vi "1_VisualAD_Train_Eval_Investigate.vi"(0 "NNFE_Paths":T1={"CFG"=path "D:/Ngene/GitHub/deepltk_examples/3_Image_Processing/36_Anomaly_Detection/NNFE/WRN_50_2_2_L3/WRN_50_2_2_BBoneL3.cfg", "BIN"=path "D:/Ngene/GitHub/deepltk_examples/3_Image_Processing/36_Anomaly_Detection/NNFE/WRN_50_2_2_L3/WRN_50_2_2_BBoneL3.bin"}, 1 "Dest. Path":path=path "D:/Ngene/GitHub/deepltk_examples/3_Image_Processing/36_Anomaly_Detection/Models", 2 "Dataset_Path(Train)":path=path "D:/Ngene/GitHub/deepltk_examples/3_Image_Processing/36_Anomaly_Detection/Dataset/Playing_Cards_3ofHearts/train", 3 "Dataset_Path(Validation)":path=path "D:/Ngene/GitHub/deepltk_examples/3_Image_Processing/36_Anomaly_Detection/Dataset/Playing_Cards_3ofHearts/test", 4 "Ground_Truth_Folder_Path":path, 5 "error in":errorcluster, 6 "NNFE CFG":T7={"Name"="Cards_3ofHearts", "Layer_Selection_By"=enum."Stride", "Feature_Layers"={"[LayerID, PatchSize]"=[{"Layer_ID"=8, "Patch_Size"=3}]}, "Interpolation_Type"=enum."Bi-Linear"}, 7 "Dim_Reduction":T11={"Method"=enum."None", "Target_Dim"=-1, "Seed"=42}, 8 "NNPC_Setup":T2={"Input_Dims"={"C"=3, "H"=320, "W"=320}, "mBatch"=1, "Device"=enum."GPU", "GPU Id"=0}, 9 "CoreSet_Params":T5={"Distance_Metric"=enum."Euclidean", "CoreSet_Size"=2000.0, "Start_idx"=3}) -> (11 "MemBank Size":i32=2000, 13 "dT_Total":dbl=4.467676200001733 format="%.2f", 14 "Model Paths":T1={"CFG"=path "D:/Ngene/GitHub/deepltk_examples/3_Image_Processing/36_Anomaly_Detection/Models/NNPC_Cards_3ofHearts__25_10_21__19_21_13/NNPC_Cards_3ofHearts_25_10_21__19_21_13.cfg", "BIN"=path "D:/Ngene/GitHub/deepltk_examples/3_Image_Processing/36_Anomaly_Detection/Models/NNPC_Cards_3ofHearts__25_10_21__19_21_13/NNPC_Cards_3ofHearts_25_10_21__19_21_13.bin"}, 15 "Evaluation Metrics":T13={"Evaluation_Metrics(Pixel)"={"Scores(Good)"={"X Values"=[4.812818005084992, 5.126218183040619, 5.4396183609962465, 5.753018538951874, 6.066418716907501, 6.379818894863129, 6.693219072818756, 7.006619250774383, 7.320019428730012, 7.633419606685639, 7.946819784641266, 8.260219962596892, 8.57362014055252, 8.88702031850815, 9.200420496463774, 9.513820674419403, 9.827220852375032, 10.14062103033066, 10.454021208286285, 10.767421386241914, 11.080821564197542, 11.394221742153167, 11.707621920108796, 12.021022098064424, 12.33442227602005, 12.647822453975678, 12.961222631931307, 13.274622809886932, 13.58802298784256, 13.901423165798189, 14.214823343753816, 14.528223521709442, 14.841623699665071, 15.155023877620698, 15.468424055576325, 15.781824233531953, 16.095224411487578, 16.408624589443207, 16.722024767398835, 17.035424945354464, 17.348825123310093, 17.662225301265718, 17.975625479221343, 18.28902565717697, 18.6024258351326, 18.91582601308823, 19.229226191043857, 19.542626368999485, 19.856026546955107, 20.169426724910736, 20.482826902866364, 20.796227080821993, 21.10962725877762, 21.423027436733246, 21.736427614688875, 22.0498277926445, 22.36322797060013, 22.676628148555757, 22.990028326511386, 23.303428504467014, 23.61682868242264, 23.930228860378268, 24.243629038333893, 24.55702921628952, 24.87042939424515, 25.18382957220078, 25.497229750156404, 25.810629928112032, 26.124030106067657, 26.437430284023286, 26.750830461978914, 27.064230639934543, 27.37763081789017, 27.691030995845797, 28.004431173801425, 28.31783135175705, 28.63123152971268, 28.944631707668307, 29.258031885623936, 29.57143206357956, 29.88483224153519, 30.198232419490814, 30.511632597446443, 30.82503277540207, 31.1384329533577, 31.451833131313325, 31.765233309268954, 32.07863348722458, 32.39203366518021, 32.705433843135836, 33.018834021091465, 33.33223419904709, 33.64563437700272, 33.95903455495835, 34.27243473291398, 34.5858349108696, 34.89923508882523, 35.21263526678085, 35.52603544473648, 35.83943562269211], "Histogram: h(x)"=[12, 30, 25, 59, 59, 56, 104, 127, 209, 665, 1209, 1807, 1859, 2067, 2834, 3589, 5408, 7210, 6807, 4828, 4040, 4505, 5906, 7156, 6805, 5885, 5510, 7034, 8552, 10101, 11654, 13725, 17151, 20990, 27298, 34167, 43115, 55164, 67689, 83371, 100999, 118723, 140188, 163813, 184123, 207176, 225854, 231272, 209192, 173806, 123606, 81028, 49666, 28142, 16542, 9622, 6023, 3610, 2523, 1694, 1329, 813, 474, 301, 185, 155, 131, 81, 73, 56, 18, 0, 0, 0, 0, 0, 0, 0, 0, 0, 0, 0, 0, 0, 0, 0, 0, 0, 0, 0, 0, 0, 0, 0, 0, 0, 0, 0, 0, 0]}, "Scores(Bad)"={"X Values"=[4.812818005084992, 5.126218183040619, 5.4396183609962465, 5.753018538951874, 6.066418716907501, 6.379818894863129, 6.693219072818756, 7.006619250774383, 7.320019428730012, 7.633419606685639, 7.946819784641266, 8.260219962596892, 8.57362014055252, 8.88702031850815, 9.200420496463774, 9.513820674419403, 9.827220852375032, 10.14062103033066, 10.454021208286285, 10.767421386241914, 11.080821564197542, 11.394221742153167, 11.707621920108796, 12.021022098064424, 12.33442227602005, 12.647822453975678, 12.961222631931307, 13.274622809886932, 13.58802298784256, 13.901423165798189, 14.214823343753816, 14.528223521709442, 14.841623699665071, 15.155023877620698, 15.468424055576325, 15.781824233531953, 16.095224411487578, 16.408624589443207, 16.722024767398835, 17.035424945354464, 17.348825123310093, 17.662225301265718, 17.975625479221343, 18.28902565717697, 18.6024258351326, 18.91582601308823, 19.229226191043857, 19.542626368999485, 19.856026546955107, 20.169426724910736, 20.482826902866364, 20.796227080821993, 21.10962725877762, 21.423027436733246, 21.736427614688875, 22.0498277926445, 22.36322797060013, 22.676628148555757, 22.990028326511386, 23.303428504467014, 23.61682868242264, 23.930228860378268, 24.243629038333893, 24.55702921628952, 24.87042939424515, 25.18382957220078, 25.497229750156404, 25.810629928112032, 26.124030106067657, 26.437430284023286, 26.750830461978914, 27.064230639934543, 27.37763081789017, 27.691030995845797, 28.004431173801425, 28.31783135175705, 28.63123152971268, 28.944631707668307, 29.258031885623936, 29.57143206357956, 29.88483224153519, 30.198232419490814, 30.511632597446443, 30.82503277540207, 31.1384329533577, 31.451833131313325, 31.765233309268954, 32.07863348722458, 32.39203366518021, 32.705433843135836, 33.018834021091465, 33.33223419904709, 33.64563437700272, 33.95903455495835, 34.27243473291398, 34.5858349108696, 34.89923508882523, 35.21263526678085, 35.52603544473648, 35.83943562269211], "Histogram: h(x)"=[2, 13, 29, 46, 40, 46, 98, 67, 82, 187, 439, 843, 1730, 1946, 2061, 2889, 3239, 5015, 7107, 6678, 4979, 3834, 4120, 5381, 6725, 6513, 5371, 4861, 5346, 6268, 6793, 6343, 6391, 6537, 6984, 7649, 7934, 8365, 9246, 10683, 12950, 16909, 22039, 29304, 40839, 56110, 76521, 98504, 120889, 138875, 144236, 138041, 125336, 103462, 82732, 70694, 63726, 59841, 58460, 58690, 59945, 62340, 65906, 70748, 73026, 73563, 70200, 64824, 55152, 46516, 38489, 31628, 25159, 20530, 16708, 14128, 11847, 10648, 9150, 8164, 7555, 6713, 5928, 5288, 4687, 4077, 3298, 2897, 2355, 2013, 1678, 1169, 900, 661, 484, 266, 150, 87, 62, 23]}, "Eval Stats"={"Scores(Good)"={"Min"=4.656118, "Max"=26.70085}, "Scores(Bad)"={"Min"=4.903742, "Max"=35.996136}, "# of Samples(Good)"=2560000, "# of Samples(Bad)"=2560000, "AUROC"=-1.0, "F1_Max"=-1.0, "Thrshld(F1_Max)"=26.70085, "Prec.(F1_Max)"=-1.0, "Recall(F1_Max)"=-1.0, "FPR(F1_Max)"=-1.0, "FNR(F1_Max)"=-1.0}}, "Evaluation_Metrics(Image)"={"Scores(Good)"={"X Values"=[23.68446270942688, 23.834939489364622, 23.98541626930237, 24.13589304924011, 24.286369829177858, 24.436846609115598, 24.587323389053346, 24.737800168991086, 24.888276948928834, 25.038753728866574, 25.18923050880432, 25.339707288742062, 25.49018406867981, 25.640660848617554, 25.791137628555298, 25.941614408493045, 26.092091188430786, 26.242567968368533, 26.393044748306274, 26.54352152824402, 26.69399830818176, 26.84447508811951, 26.99495186805725, 27.145428647994997, 27.295905427932738, 27.446382207870485, 27.596858987808226, 27.747335767745973, 27.897812547683714, 28.04828932762146, 28.1987661075592, 28.34924288749695, 28.49971966743469, 28.650196447372437, 28.800673227310178, 28.951150007247925, 29.10162678718567, 29.252103567123413, 29.402580347061157, 29.5530571269989, 29.703533906936645, 29.85401068687439, 30.004487466812137, 30.154964246749877, 30.305441026687625, 30.455917806625365, 30.606394586563113, 30.756871366500853, 30.9073481464386, 31.05782492637634, 31.20830170631409, 31.35877848625183, 31.509255266189577, 31.659732046127317, 31.810208826065065, 31.960685606002805, 32.111162385940546, 32.26163916587829, 32.41211594581604, 32.56259272575379, 32.71306950569153, 32.86354628562927, 33.01402306556702, 33.164499845504764, 33.314976625442505, 33.465453405380245, 33.61593018531799, 33.76640696525574, 33.91688374519348, 34.06736052513122, 34.21783730506897, 34.368314085006716, 34.518790864944464, 34.6692676448822, 34.819744424819945, 34.97022120475769, 35.12069798469544, 35.27117476463317, 35.42165154457092, 35.57212832450867, 35.722605104446416, 35.87308188438415, 36.0235586643219, 36.174035444259644, 36.32451222419739, 36.47498900413513, 36.62546578407287, 36.77594256401062, 36.92641934394837, 37.07689612388611, 37.22737290382385, 37.377849683761596, 37.528326463699344, 37.678803243637084, 37.829280023574825, 37.97975680351257, 38.13023358345032, 38.28071036338807, 38.4311871433258, 38.58166392326355], "Histogram: h(x)"=[1, 1, 0, 0, 0, 0, 1, 1, 0, 2, 2, 3, 2, 1, 1, 1, 0, 0, 0, 2, 0, 0, 0, 0, 0, 0, 0, 0, 0, 0, 0, 0, 0, 0, 1, 0, 2, 1, 0, 1, 0, 0, 0, 0, 0, 0, 0, 0, 0, 0, 0, 0, 0, 0, 1, 0, 0, 0, 0, 1, 0, 0, 0, 0, 0, 0, 0, 0, 0, 0, 0, 0, 0, 0, 0, 0, 0, 0, 0, 0, 0, 0, 0, 0, 0, 0, 0, 0, 0, 0, 0, 0, 0, 0, 0, 0, 0, 0, 0, 0]}, "Scores(Bad)"={"X Values"=[23.68446270942688, 23.834939489364622, 23.98541626930237, 24.13589304924011, 24.286369829177858, 24.436846609115598, 24.587323389053346, 24.737800168991086, 24.888276948928834, 25.038753728866574, 25.18923050880432, 25.339707288742062, 25.49018406867981, 25.640660848617554, 25.791137628555298, 25.941614408493045, 26.092091188430786, 26.242567968368533, 26.393044748306274, 26.54352152824402, 26.69399830818176, 26.84447508811951, 26.99495186805725, 27.145428647994997, 27.295905427932738, 27.446382207870485, 27.596858987808226, 27.747335767745973, 27.897812547683714, 28.04828932762146, 28.1987661075592, 28.34924288749695, 28.49971966743469, 28.650196447372437, 28.800673227310178, 28.951150007247925, 29.10162678718567, 29.252103567123413, 29.402580347061157, 29.5530571269989, 29.703533906936645, 29.85401068687439, 30.004487466812137, 30.154964246749877, 30.305441026687625, 30.455917806625365, 30.606394586563113, 30.756871366500853, 30.9073481464386, 31.05782492637634, 31.20830170631409, 31.35877848625183, 31.509255266189577, 31.659732046127317, 31.810208826065065, 31.960685606002805, 32.111162385940546, 32.26163916587829, 32.41211594581604, 32.56259272575379, 32.71306950569153, 32.86354628562927, 33.01402306556702, 33.164499845504764, 33.314976625442505, 33.465453405380245, 33.61593018531799, 33.76640696525574, 33.91688374519348, 34.06736052513122, 34.21783730506897, 34.368314085006716, 34.518790864944464, 34.6692676448822, 34.819744424819945, 34.97022120475769, 35.12069798469544, 35.27117476463317, 35.42165154457092, 35.57212832450867, 35.722605104446416, 35.87308188438415, 36.0235586643219, 36.174035444259644, 36.32451222419739, 36.47498900413513, 36.62546578407287, 36.77594256401062, 36.92641934394837, 37.07689612388611, 37.22737290382385, 37.377849683761596, 37.528326463699344, 37.678803243637084, 37.829280023574825, 37.97975680351257, 38.13023358345032, 38.28071036338807, 38.4311871433258, 38.58166392326355], "Histogram: h(x)"=[0, 0, 0, 0, 0, 0, 0, 0, 0, 0, 0, 0, 0, 0, 0, 0, 0, 0, 0, 0, 0, 0, 0, 0, 0, 0, 0, 0, 0, 0, 0, 0, 0, 0, 0, 0, 0, 0, 0, 0, 0, 0, 0, 0, 0, 0, 0, 0, 0, 0, 0, 0, 0, 0, 0, 0, 0, 0, 0, 0, 0, 0, 0, 0, 0, 0, 0, 0, 0, 0, 0, 0, 0, 0, 0, 1, 0, 1, 0, 0, 1, 0, 0, 1, 1, 1, 2, 4, 1, 1, 1, 1, 1, 0, 1, 1, 3, 1, 1, 1]}, "Eval Stats"={"Scores(Good)"={"Min"=23.609224, "Max"=32.612473}, "Scores(Bad)"={"Min"=34.950077, "Max"=38.656902}, "# of Samples(Good)"=25, "# of Samples(Bad)"=25, "AUROC"=1.0878985, "F1_Max"=-1.0, "Thrshld(F1_Max)"=33.781273, "Prec.(F1_Max)"=-1.0, "Recall(F1_Max)"=-1.0, "FPR(F1_Max)"=-1.0, "FNR(F1_Max)"=-1.0}}} {"Evaluation_Metrics(Image)"."Eval Stats"."Recall(F1_Max)" format="%#.5f"; "Evaluation_Metrics(Image)"."Eval Stats"."FPR(F1_Max)" format="%#.5f"; "Evaluation_Metrics(Image)"."Eval Stats"."FNR(F1_Max)" format="%#.5f"; "Evaluation_Metrics(Image)"."Eval Stats"."Prec.(F1_Max)" format="%#.5f"; "Evaluation_Metrics(Image)"."Eval Stats"."F1_Max" format="%#.5f"; "Evaluation_Metrics(Image)"."Eval Stats"."AUROC" format="%#.5f"; "Evaluation_Metrics(Image)"."Eval Stats"."Scores(Bad)"."Min" format="%#_5g"; "Evaluation_Metrics(Image)"."Eval Stats"."Scores(Good)"."Min" format="%#_5g"; "Evaluation_Metrics(Image)"."Eval Stats"."Thrshld(F1_Max)" format="%#_5f"; "Evaluation_Metrics(Pixel)"."Eval Stats"."Recall(F1_Max)" format="%#.5f"; "Evaluation_Metrics(Pixel)"."Eval Stats"."FPR(F1_Max)" format="%#.5f"; "Evaluation_Metrics(Pixel)"."Eval Stats"."FNR(F1_Max)" format="%#.5f"; "Evaluation_Metrics(Pixel)"."Eval Stats"."Prec.(F1_Max)" format="%#.5f"; "Evaluation_Metrics(Pixel)"."Eval Stats"."F1_Max" format="%#.5f"; "Evaluation_Metrics(Pixel)"."Eval Stats"."AUROC" format="%#.5f"; "Evaluation_Metrics(Pixel)"."Eval Stats"."Scores(Bad)"."Min" format="%#_5g"; "Evaluation_Metrics(Pixel)"."Eval Stats"."Scores(Good)"."Min" format="%#_5g"; "Evaluation_Metrics(Pixel)"."Eval Stats"."Thrshld(F1_Max)" format="%#_5f"}, 18 "Dataset Size":i32=50)   [LabVIEW 2020]
uses:
  <vilib>/Ngene/DeepLTK Anomaly Detection Addon/Toolkit/API/Controls/NN_Paths.ctl
  <vilib>/Ngene/DeepLTK Anomaly Detection Addon/Toolkit/API/Controls/NNPC_Setup.ctl
  <vilib>/Ngene/Deep Learning Toolkit/Toolkit/NN_Data/API/NN_Dims(C,H,W).ctl
  <vilib>/Ngene/Deep Learning Toolkit/Toolkit/NN_Network/Controls/NN_Device.ctl
  <vilib>/Ngene/DeepLTK Anomaly Detection Addon/Toolkit/API/Controls/NNPC_Coreset_Params.ctl
  <vilib>/Ngene/DeepLTK Anomaly Detection Addon/Toolkit/API/Controls/Distance_Metric.ctl
  <vilib>/Ngene/DeepLTK Anomaly Detection Addon/Toolkit/API/Controls/NNFE_CFG.ctl
  <vilib>/Ngene/DeepLTK Anomaly Detection Addon/Toolkit/API/Controls/Layer_Selector.ctl
  <vilib>/Ngene/DeepLTK Anomaly Detection Addon/Toolkit/API/Controls/Feature_Layer_Selector.ctl
  <vilib>/Ngene/DeepLTK Anomaly Detection Addon/Toolkit/API/Controls/Interpolation_Selector.ctl
  <vilib>/Ngene/DeepLTK Anomaly Detection Addon/Toolkit/API/Controls/NNPC_Random_Projection_CFG.ctl
  <vilib>/Ngene/DeepLTK Anomaly Detection Addon/Toolkit/API/Controls/Dim_Reduction_Method.ctl
  <vilib>/Ngene/DeepLTK Anomaly Detection Addon/Toolkit/API/Controls/Evaluation_Metrics(Pixel_Image).ctl
  <vilib>/Ngene/DeepLTK Anomaly Detection Addon/Toolkit/API/Controls/Evaluation_Metrics.ctl
  <vilib>/Ngene/DeepLTK Anomaly Detection Addon/Toolkit/API/Controls/Eval_Results.ctl
  <vilib>/Ngene/DeepLTK Anomaly Detection Addon/Toolkit/API/Controls/MinMax.ctl
  subVIs/Feature_Retrieval/Controls/Patch_RF_Scales.ctl
  subVIs/Dataset_Reader/Controls/Read_Options.ctl
  <vilib>/Ngene/DeepLTK Anomaly Detection Addon/Toolkit/API/Controls/NNPC_PreProcessing_Options.ctl
  <vilib>/Ngene/DeepLTK Anomaly Detection Addon/Toolkit/API/Controls/Crop_CFG.ctl
  <vilib>/Ngene/DeepLTK Anomaly Detection Addon/Toolkit/API/Controls/NNPC_DS_Stats.ctl
  <vilib>/Ngene/DeepLTK Anomaly Detection Addon/Toolkit/API/Controls/Image_Stats_RGB.ctl
  subVIs/Train_Case_Investigation/Controls/Detection_Results.ctl
  <vilib>/Ngene/DeepLTK Anomaly Detection Addon/Toolkit/API/Controls/Feature_Scorer_Params.ctl
  <vilib>/Ngene/DeepLTK Anomaly Detection Addon/Toolkit/API/Controls/Gaussian_Blur.ctl
  <vilib>/vision/Image Controls.llb/IMAQ Image.ctl
  subVIs/Visualizer/Controls/Display_Options.ctl
  subVIs/Visualizer/Controls/ROI_Display_Options.ctl
  subVIs/Visualizer/Controls/Heatmap_Display_Options.ctl
  subVIs/Visualizer/Controls/ColorMap.ctl
  subVIs/Visualizer/Controls/Report_Images_CFG.ctl
  <vilib>/Ngene/CuLab - GPU Accelerated Toolkit/Toolkit/Low_Level/Tensor_Classes/T_Children/T2D/T2D_Children/T2D_SGL/T2D_SGL.lvclass
  subVIs/Feature_Retrieval/Controls/Dims(2D)ctl.ctl
  4cc6689b-300a-41eb-b37a-9ba3a5a9262f.vi
  f46c6ce4-2999-47cd-b61f-bf4da423de8f.vi
  <vilib>/Utility/High Resolution Relative Seconds.vi
  <vilib>/Ngene/DeepLTK Anomaly Detection Addon/Toolkit/API/NNPC_Predict/NNPC_Predict(Dataset).vi
  <vilib>/Ngene/DeepLTK Anomaly Detection Addon/Toolkit/API/NNPC_Predict/NNPC_Predict(Single).vi
  <vilib>/Ngene/Deep Learning Toolkit/Toolkit/NN_Data/subVIs/Get_Data_Vals/2D/NN_Data_Get_ValByRef(2D_SGL).vi
  <vilib>/Ngene/CuLab - GPU Accelerated Toolkit/Toolkit/Low_Level/Tensor_Classes/T_Children/T2D/T2D_Children/T2D_SGL/Pull.vi
  <vilib>/Ngene/DeepLTK Anomaly Detection Addon/Toolkit/DeepLTK_Anomaly_Detection_Addon.lvlib
  <vilib>/Ngene/Deep Learning Toolkit/Toolkit/Deep_Learning_Toolkit_by_Ngene.lvlib
  <vilib>/Ngene/CuLab - GPU Accelerated Toolkit/Toolkit/CuLab.lvlib
  <vilib>/ptbypt/NI_PtbyPt.lvlib
  <vilib>/vision/NI_Vision_Development_Module.lvlib
panel:
  out "Last Mouse Position:All Elements":cluster{"X":i32, "Y":i32}={"X"=160, "Y"=149}
  in  "?":enum32{"Train Eval", "Investigation"}(tab)=enum."Investigation"
  out "dT_Gen_Embed":dbl=0.13866830000188202 format="%.2f"
  out "dT_Coreset":dbl=0.930330999995931 format="%.2f"
  out "Coreset_Max_Distances":sgl[](graph)=[74.63289, 72.04883, 65.9075, 60.996574, 60.18411, 59.513584, 58.878304, 56.79366, 54.17582, 53.42479, 52.945797, 52.372814, 52.115356, 51.732815, 51.65042, 51.541634, 51.26071, 49.480553, 49.472836, 49.072372, 48.75653, 48.561096, 48.094997, 47.537315, 47.519333, 47.487957, 47.22181, 46.51589, 46.2671, 45.79364, 45.73255, 45.532997, 45.391308, 45.316776, 45.271545, 45.25147, 45.156315, 45.14392, 44.677746, 44.659378, 44.512352, 44.004093, 43.96949, 43.823536, 43.820038, 43.80221, 43.662075, 43.425877, 43.2432, 43.23487, 42.94812, 42.740986, 42.370102, 42.342667, 42.31884, 42.13516, 41.964935, 41.87032, 41.85968, 41.571934, 41.54662, 41.416203, 41.402004, 41.35856, 41.254498, 41.21967, 41.185936, 41.024414, 40.920685, 40.905533, 40.766216, 40.750626, 40.60767, 40.563248, 40.53888, 40.36831, 40.33242, 40.122494, 40.079067, 39.94822, 39.87803, 39.872265, 39.868748, 39.822437, 39.815388, 39.680523, 39.41898, 39.2283, 39.13182, 39.122597, 39.068485, 39.03738, 38.999065, 38.998318, 38.957848, 38.83956, 38.83068, 38.780052, 38.777523, 38.69353, 38.679825, 38.55367, 38.553055, 38.531246, 38.489243, 38.38429, 38.27287, 38.25715, 38.1597, 38.077477, 38.011055, 37.98357, 37.926243, 37.834633, 37.803535, 37.754963, 37.73896, 37.734123, 37.72009, 37.681293, 37.65433, 37.619587, 37.558743, 37.52339, 37.51869, 37.480705, 37.47731, 37.463604, 37.46054, 37.407772, 37.28176, 37.072742, 37.051327, 37.035007, 37.014065, 36.95656, 36.83368, 36.805695, 36.78203, 36.775135, 36.744053, 36.69711, 36.679565, 36.643654, 36.639763, 36.638096, 36.55906, 36.54673, 36.495243, 36.482605, 36.445538, 36.424606, 36.396915, 36.379086, 36.336227, 36.32822, 36.314766, 36.312244, 36.2889, 36.273247, 36.267826, 36.233395, 36.23158, 36.058594, 36.02851, 35.997612, 35.983593, 35.972218, 35.876522, 35.857983, 35.77934, 35.777756, 35.740387, 35.726856, 35.695038, 35.665398, 35.664574, 35.616722, 35.574505, 35.517628, 35.50664, 35.454994, 35.453636, 35.450985, 35.43546, 35.361816, 35.31139, 35.303192, 35.262367, 35.2567, 35.204647, 35.101616, 35.099037, 35.052883, 34.983032, 34.963627, 34.937862, 34.93076, 34.90355, 34.882656, 34.796406, 34.76938, 34.726673, 34.64066, 34.614296, 34.59488, 34.586716, 34.55041, 34.540695, 34.493084, 34.47748, 34.477425, 34.46085, 34.45067, 34.41504, 34.409966, 34.361023, 34.3604, 34.357227, 34.35542, 34.28918, 34.27293, 34.252075, 34.248764, 34.209614, 34.205414, 34.192482, 34.187737, 34.16094, 34.119316, 34.111725, 34.058525, 34.047394, 34.041836, 34.02031, 33.94235, 33.921303, 33.917324, 33.895557, 33.87933, 33.85728, 33.826424, 33.806484, 33.78179, 33.743397, 33.734467, 33.727722, 33.71431, 33.71039, 33.70629, 33.68326, 33.679527, 33.679424, 33.634922, 33.63319, 33.60709, 33.544888, 33.529297, 33.522717, 33.51942, 33.47897, 33.475685, 33.42354, 33.405952, 33.392845, 33.38609, 33.371647, 33.3662, 33.351658, 33.29621, 33.275784, 33.247925, 33.246975, 33.198704, 33.18313, 33.171215, 33.1478, 33.13651, 33.12186, 33.105537, 33.101887, 33.088806, 33.08757, 33.081383, 33.07139, 33.044952, 33.044094, 33.032417, 33.00067, 32.895134, 32.885048, 32.87759, 32.876476, 32.85487, 32.846233, 32.81955, 32.77868, 32.7757, 32.746307, 32.735138, 32.69302, 32.68806, 32.683025, 32.67158, 32.66998, 32.656265, 32.651375, 32.640472, 32.632706, 32.58497, 32.539818, 32.537, 32.53454, 32.511257, 32.474903, 32.444187, 32.40475, 32.39956, 32.36942, 32.3373, 32.335167, 32.328564, 32.32187, 32.31347, 32.3072, 32.298923, 32.285694, 32.2609, 32.23464, 32.205917, 32.18647, 32.186, 32.16417, 32.152065, 32.13823, 32.053696, 32.041653, 32.02521, 32.014492, 32.01189, 32.00962, 31.998943, 31.962082, 31.908989, 31.894564, 31.887466, 31.87752, 31.875046, 31.867075, 31.834318, 31.807188, 31.801746, 31.7938, 31.790014, 31.787863, 31.751669, 31.749931, 31.717865, 31.710321, 31.694387, 31.693163, 31.689518, 31.650997, 31.639025, 31.626057, 31.625177, 31.624332, 31.613426, 31.612322, 31.605864, 31.605, 31.593124, 31.567505, 31.54225, 31.541313, 31.492598, 31.469294, 31.467411, 31.463928, 31.426626, 31.410044, 31.404673, 31.402176, 31.397316, 31.34294, 31.331583, 31.31381, 31.308102, 31.25104, 31.243008, 31.241499, 31.233292, 31.20662, 31.199451, 31.184141, 31.179012, 31.178108, 31.152035, 31.147362, 31.141657, 31.138166, 31.137033, 31.108398, 31.105356, 31.08858, 31.083738, 31.076942, 31.059608, 31.057682, 31.05663, 31.05289, 31.041979, 31.040327, 31.016783, 31.007504, 30.997574, 30.996416, 30.994896, 30.980762, 30.961315, 30.941713, 30.935282, 30.922916, 30.90964, 30.897049, 30.891487, 30.86979, 30.85223, 30.84033, 30.833637, 30.823944, 30.783503, 30.773739, 30.755224, 30.752024, 30.7446, 30.724556, 30.717562, 30.713154, 30.700043, 30.693228, 30.676443, 30.659563, 30.658257, 30.63746, 30.60626, 30.593023, 30.572891, 30.559488, 30.520845, 30.51281, 30.50892, 30.484852, 30.46742, 30.447424, 30.441519, 30.420145, 30.412685, 30.403616, 30.392235, 30.385174, 30.36222, 30.3521, 30.327614, 30.323336, 30.30007, 30.294832, 30.254116, 30.248281, 30.245504, 30.236834, 30.236761, 30.229488, 30.224348, 30.220875, 30.196548, 30.175112, 30.169064, 30.164232, 30.16182, 30.153303, 30.151367, 30.147991, 30.146793, 30.143982, 30.135817, 30.117826, 30.110044, 30.108612, 30.099274, 30.089037, 30.07584, 30.067787, 30.060932, 30.060194, 30.054358, 30.038467, 30.036907, 30.031218, 30.024559, 30.021517, 30.012909, 30.00926, 30.008177, 29.996866, 29.995646, 29.973492, 29.965368, 29.936995, 29.931097, 29.916052, 29.875217, 29.867563, 29.85808, 29.854513, 29.840591, 29.83974, 29.80229, 29.789534, 29.733944, 29.715965, 29.700405, 29.691763, 29.688778, 29.666502, 29.666103, 29.634409, 29.619272, 29.599186, 29.59578, 29.592995, 29.591555, 29.565662, 29.56544, 29.559654, 29.548986, 29.527737, 29.523722, 29.51594, 29.506409, 29.50609, 29.505892, 29.498882, 29.49048, 29.464085, 29.459055, 29.458101, 29.453644, 29.453207, 29.427757, 29.418444, 29.418087, 29.41232, 29.404041, 29.399662, 29.378332, 29.376192, 29.36918, 29.34554, 29.341112, 29.328203, 29.323118, 29.309168, 29.30597, 29.298103, 29.295399, 29.289637, 29.264795, 29.256285, 29.255024, 29.24869, 29.246862, 29.234747, 29.231247, 29.226963, 29.209942, 29.206774, 29.206657, 29.182213, 29.162693, 29.155941, 29.150087, 29.149412, 29.147745, 29.14759, 29.14225, 29.13918, 29.135572, 29.111744, 29.085903, 29.073553, 29.061829, 29.060333, 29.043554, 29.036531, 29.016033, 29.004719, 28.992052, 28.97764, 28.971266, 28.96344, 28.95987, 28.954689, 28.917282, 28.8915, 28.88052, 28.878534, 28.871973, 28.871592, 28.86475, 28.8486, 28.843124, 28.843004, 28.839191, 28.825758, 28.821184, 28.81173, 28.80448, 28.802704, 28.7947, 28.79013, 28.777992, 28.767895, 28.764105, 28.755354, 28.754517, 28.741074, 28.731506, 28.728474, 28.719986, 28.706642, 28.703724, 28.69818, 28.695814, 28.685104, 28.677992, 28.676477, 28.668686, 28.66531, 28.63774, 28.633732, 28.621542, 28.613997, 28.60804, 28.598135, 28.598019, 28.59533, 28.579266, 28.56232, 28.558256, 28.542568, 28.524591, 28.523787, 28.518839, 28.511349, 28.498951, 28.494705, 28.49342, 28.488644, 28.45741, 28.43258, 28.426233, 28.419994, 28.414469, 28.40276, 28.40242, 28.398857, 28.390207, 28.388626, 28.38595, 28.384506, 28.378815, 28.374853, 28.342592, 28.341658, 28.318579, 28.292746, 28.283567, 28.272017, 28.270592, 28.265728, 28.263626, 28.245527, 28.22971, 28.214657, 28.210331, 28.201588, 28.190601, 28.188604, 28.185534, 28.180449, 28.174246, 28.16436, 28.161045, 28.143814, 28.141817, 28.127739, 28.125708, 28.121723, 28.120676, 28.11308, 28.11308, 28.103811, 28.101274, 28.089613, 28.054504, 28.054338, 28.054321, 28.046505, 28.045534, 28.02131, 28.021101, 28.010326, 27.989527, 27.988358, 27.987564, 27.987528, 27.971308, 27.942131, 27.940392, 27.938164, 27.936512, 27.930643, 27.926744, 27.925167, 27.923698, 27.9216, 27.919703, 27.91947, 27.913221, 27.903416, 27.894821, 27.869053, 27.866884, 27.86174, 27.860912, 27.860071, 27.858574, 27.85051, 27.84461, 27.840843, 27.838436, 27.837217, 27.835857, 27.828554, 27.815067, 27.809696, 27.805714, 27.786892, 27.769876, 27.75847, 27.755142, 27.750929, 27.70976, 27.703085, 27.700565, 27.694818, 27.693521, 27.69339, 27.68676, 27.68674, 27.6843, 27.679413, 27.678804, 27.678556, 27.673326, 27.66865, 27.666246, 27.664732, 27.659525, 27.652538, 27.647669, 27.636465, 27.627687, 27.626883, 27.613623, 27.612549, 27.605974, 27.577944, 27.570196, 27.554146, 27.539318, 27.53196, 27.530708, 27.52541, 27.52216, 27.521193, 27.51168, 27.508318, 27.500643, 27.492365, 27.470976, 27.461737, 27.458313, 27.452303, 27.451332, 27.450466, 27.450008, 27.447535, 27.442247, 27.438034, 27.413359, 27.393433, 27.391388, 27.390345, 27.389114, 27.38874, 27.38336, 27.370367, 27.364555, 27.362154, 27.359272, 27.357946, 27.35515, 27.345987, 27.34404, 27.339867, 27.334686, 27.321741, 27.316103, 27.313545, 27.312643, 27.303637, 27.289217, 27.288336, 27.280802, 27.2787, 27.27187, 27.255634, 27.251379, 27.250444, 27.241856, 27.23333, 27.223566, 27.221056, 27.216818, 27.205637, 27.201406, 27.198238, 27.179758, 27.165724, 27.163666, 27.161366, 27.157661, 27.154272, 27.152987, 27.15072, 27.149183, 27.135857, 27.13219, 27.129387, 27.123106, 27.119041, 27.106632, 27.104723, 27.10439, 27.093876, 27.089867, 27.086098, 27.085157, 27.077679, 27.073847, 27.07224, 27.069302, 27.05738, 27.042162, 27.03406, 27.033756, 27.033003, 27.028202, 27.028011, 27.026241, 27.02603, 27.008364, 27.007322, 27.005285, 26.998526, 26.996456, 26.975739, 26.96808, 26.967669, 26.965935, 26.96166, 26.95567, 26.944332, 26.934599, 26.922106, 26.921925, 26.916183, 26.912048, 26.904398, 26.898283, 26.88461, 26.874727, 26.857452, 26.853962, 26.852688, 26.847748, 26.845833, 26.843178, 26.840658, 26.83872, 26.832214, 26.829868, 26.829222, 26.828884, 26.820175, 26.814976, 26.809359, 26.80816, 26.798237, 26.780275, 26.778042, 26.771595, 26.763327, 26.758905, 26.756968, 26.746494, 26.730179, 26.72742, 26.726803, 26.719765, 26.71802, 26.712418, 26.702742, 26.700232, 26.69317, 26.690958, 26.68365, 26.673298, 26.670246, 26.664904, 26.645788, 26.64556, 26.645151, 26.631098, 26.625101, 26.623213, 26.61754, 26.61697, 26.61372, 26.611177, 26.61015, 26.604296, 26.603516, 26.595127, 26.58584, 26.584852, 26.579773, 26.579416, 26.574635, 26.57272, 26.566921, 26.566525, 26.543678, 26.525787, 26.523703, 26.518677, 26.512665, 26.50946, 26.501478, 26.497734, 26.497084, 26.476257, 26.46969, 26.461536, 26.45904, 26.457355, 26.455114, 26.451754, 26.445044, 26.437214, 26.432144, 26.43026, 26.43026, 26.429174, 26.41065, 26.409061, 26.401127, 26.391582, 26.389528, 26.38758, 26.377764, 26.376045, 26.368353, 26.365261, 26.353933, 26.346493, 26.342953, 26.342657, 26.337513, 26.33317, 26.33297, 26.306765, 26.306728, 26.29539, 26.292887, 26.28446, 26.273872, 26.273413, 26.26073, 26.257719, 26.252028, 26.251776, 26.24614, 26.245153, 26.242777, 26.24274, 26.233952, 26.231178, 26.208948, 26.205719, 26.19387, 26.19161, 26.190922, 26.190529, 26.18805, 26.182484, 26.180143, 26.177551, 26.166403, 26.166216, 26.161682, 26.160841, 26.158714, 26.155018, 26.122557, 26.11205, 26.10291, 26.102076, 26.096584, 26.094658, 26.091831, 26.088463, 26.084785, 26.083456, 26.073397, 26.072527, 26.070864, 26.06696, 26.064785, 26.055994, 26.03999, 26.0378, 26.034542, 26.032545, 26.025612, 26.02489, 26.024252, 26.022142, 26.016628, 26.012054, 26.008299, 26.004713, 26.001005, 25.99662, 25.99134, 25.97815, 25.978075, 25.97783, 25.973835, 25.973, 25.971565, 25.968792, 25.963099, 25.962591, 25.953215, 25.95234, 25.943668, 25.94088, 25.940248, 25.930624, 25.926975, 25.92686, 25.91463, 25.91392, 25.912169, 25.908606, 25.895004, 25.883982, 25.875849, 25.873693, 25.872272, 25.864502, 25.858133, 25.855026, 25.853941, 25.85092, 25.850306, 25.845846, 25.835804, 25.834045, 25.831882, 25.829868, 25.828339, 25.820992, 25.803276, 25.802282, 25.796984, 25.794329, 25.79158, 25.784218, 25.78304, 25.776808, 25.77675, 25.775269, 25.774895, 25.77158, 25.768017, 25.76671, 25.7619, 25.760574, 25.757498, 25.756939, 25.744776, 25.743116, 25.736837, 25.735128, 25.728876, 25.724943, 25.723192, 25.719994, 25.715342, 25.713537, 25.709606, 25.708391, 25.706871, 25.688332, 25.687828, 25.6852, 25.67594, 25.675331, 25.66742, 25.66485, 25.664595, 25.660189, 25.657526, 25.651701, 25.65103, 25.650068, 25.649769, 25.633068, 25.6282, 25.62438, 25.620655, 25.620378, 25.611092, 25.610323, 25.598728, 25.59531, 25.59394, 25.586987, 25.580683, 25.580334, 25.574265, 25.56802, 25.565737, 25.560629, 25.558908, 25.556396, 25.553865, 25.545818, 25.5419, 25.534721, 25.528831, 25.524794, 25.516462, 25.512701, 25.508327, 25.50703, 25.49897, 25.497673, 25.482157, 25.46831, 25.467524, 25.458864, 25.455173, 25.451124, 25.450838, 25.45006, 25.44959, 25.44885, 25.443518, 25.43976, 25.423758, 25.419834, 25.417, 25.416742, 25.41618, 25.415224, 25.409075, 25.39908, 25.398455, 25.392889, 25.391043, 25.389477, 25.388744, 25.387125, 25.3835, 25.379902, 25.379513, 25.374615, 25.363934, 25.35657, 25.355865, 25.353642, 25.352486, 25.346668, 25.346096, 25.344376, 25.342276, 25.334057, 25.331778, 25.325787, 25.324564, 25.318132, 25.315027, 25.28874, 25.288357, 25.287777, 25.283964, 25.282656, 25.281149, 25.27815, 25.276913, 25.27109, 25.25785, 25.255037, 25.254206, 25.252262, 25.24824, 25.244314, 25.243095, 25.240261, 25.237417, 25.237272, 25.23706, 25.23673, 25.235405, 25.234472, 25.232492, 25.231216, 25.22826, 25.224665, 25.222971, 25.221315, 25.21859, 25.215738, 25.215385, 25.210558, 25.2093, 25.201014, 25.200417, 25.197758, 25.1971, 25.190403, 25.183786, 25.183556, 25.178188, 25.176506, 25.173616, 25.171463, 25.161926, 25.1608, 25.160637, 25.159424, 25.156658, 25.156425, 25.154745, 25.13456, 25.132423, 25.131033, 25.127012, 25.112345, 25.111937, 25.11009, 25.108437, 25.10618, 25.10604, 25.090145, 25.07201, 25.069366, 25.067087, 25.064949, 25.060776, 25.060387, 25.057327, 25.055252, 25.05491, 25.053215, 25.051685, 25.047865, 25.04732, 25.044788, 25.04109, 25.031563, 25.031294, 25.028265, 25.023094, 25.02124, 25.01948, 25.01678, 25.015785, 25.012848, 25.010994, 25.009563, 25.007954, 25.00685, 25.004501, 25.000576, 24.9937, 24.993046, 24.992195, 24.991127, 24.985474, 24.985035, 24.982573, 24.981033, 24.97941, 24.975925, 24.9733, 24.973042, 24.971546, 24.96988, 24.96917, 24.962608, 24.958227, 24.956573, 24.954569, 24.952162, 24.951075, 24.948423, 24.947142, 24.944157, 24.943823, 24.937765, 24.93656, 24.926311, 24.91511, 24.912777, 24.91068, 24.902113, 24.901829, 24.899221, 24.897152, 24.895298, 24.893965, 24.891165, 24.889748, 24.87737, 24.876173, 24.865978, 24.865213, 24.864546, 24.863926, 24.860651, 24.858065, 24.850319, 24.849546, 24.847195, 24.845018, 24.836369, 24.83164, 24.829054, 24.82718, 24.826433, 24.826233, 24.823547, 24.818914, 24.817724, 24.817192, 24.815905, 24.814861, 24.814388, 24.811712, 24.808382, 24.80817, 24.805523, 24.804922, 24.802551, 24.802147, 24.799734, 24.784615, 24.779781, 24.779053, 24.77828, 24.777714, 24.777319, 24.772558, 24.767208, 24.764624, 24.763914, 24.76214, 24.751282, 24.751213, 24.74862, 24.748604, 24.747267, 24.747139, 24.739492, 24.729927, 24.724863, 24.724424, 24.71959, 24.717976, 24.716677, 24.71183, 24.707537, 24.702028, 24.692148, 24.689062, 24.685799, 24.677738, 24.676733, 24.676422, 24.675041, 24.675016, 24.670515, 24.6691, 24.666288, 24.664427, 24.664091, 24.658121, 24.64968, 24.646257, 24.645811, 24.645082, 24.643066, 24.63954, 24.634277, 24.63358, 24.631939, 24.631428, 24.628569, 24.625198, 24.62074, 24.61747, 24.613537, 24.609499, 24.599298, 24.599007, 24.594261, 24.588856, 24.588299, 24.584774, 24.58255, 24.578209, 24.577295, 24.575035, 24.574524, 24.569118, 24.567148, 24.564825, 24.560179, 24.552677, 24.551668, 24.543468, 24.543274, 24.538797, 24.533768, 24.532175, 24.53121, 24.528612, 24.523407, 24.519264, 24.515879, 24.515242, 24.513105, 24.510246, 24.507452, 24.507284, 24.49417, 24.4939, 24.490486, 24.490198, 24.490088, 24.485178, 24.484041, 24.482725, 24.482021, 24.476017, 24.475983, 24.456015, 24.455996, 24.455816, 24.454906, 24.454798, 24.451033, 24.449125, 24.43742, 24.436651, 24.431261, 24.426298, 24.425898, 24.425098, 24.423464, 24.42172, 24.411732, 24.393843, 24.39146, 24.388178, 24.386927, 24.379538, 24.379236, 24.37804, 24.375952, 24.375675, 24.36963, 24.36458, 24.363104, 24.354519, 24.353155, 24.35087, 24.350203, 24.34693, 24.342402, 24.342245, 24.34028, 24.337542, 24.327438, 24.327276, 24.324436, 24.322529, 24.318129, 24.317862, 24.315834, 24.309446, 24.30451, 24.29666, 24.296528, 24.292599, 24.29068, 24.29049, 24.289143, 24.287422, 24.281933, 24.279892, 24.276806, 24.270359, 24.270092, 24.268295, 24.26473, 24.262964, 24.261051, 24.260931, 24.259432, 24.256542, 24.250235, 24.248983, 24.247593, 24.24693, 24.240812, 24.240475, 24.237402, 24.232935, 24.22911, 24.228703, 24.224869, 24.222282, 24.221128, 24.22004, 24.214, 24.209414, 24.207254, 24.203705, 24.196693, 24.195387, 24.193071, 24.190483, 24.190456, 24.184412, 24.179783, 24.179096, 24.178883, 24.175556, 24.17383, 24.173435, 24.170532, 24.16999, 24.161566, 24.161339, 24.157179, 24.156134, 24.156118, 24.152449, 24.148659, 24.145424, 24.140524, 24.133327, 24.131456, 24.128475, 24.128067, 24.12617, 24.121498, 24.109816, 24.105446, 24.102919, 24.100077, 24.0961, 24.09579, 24.093344, 24.091074, 24.089018, 24.08325, 24.082632, 24.081669, 24.079266, 24.076168, 24.075626, 24.071453, 24.071112, 24.071041, 24.062551, 24.061672, 24.061424, 24.060318, 24.059963, 24.05701, 24.053417, 24.050758, 24.04818, 24.04558, 24.044708, 24.04316, 24.042656, 24.039274, 24.036247, 24.031778, 24.026556, 24.024534, 24.021484, 24.019793, 24.00097, 24.00026, 24.000214, 23.997763, 23.98716, 23.987068, 23.98145, 23.977375, 23.971888, 23.970303, 23.967722, 23.966112, 23.963173, 23.96223, 23.958124, 23.956774, 23.94995, 23.948563, 23.9429, 23.941233, 23.931894, 23.931574, 23.92812, 23.923891, 23.922686, 23.9194, 23.918037, 23.9179, 23.916378, 23.916225, 23.913494, 23.911932, 23.90621, 23.90292, 23.900337, 23.897997, 23.89643, 23.894186, 23.893051, 23.890823, 23.88875, 23.883926, 23.883419, 23.879366, 23.87904, 23.874489, 23.872627, 23.871492, 23.865631, 23.86424, 23.863478, 23.858183, 23.854774, 23.850107, 23.849089, 23.840975, 23.836525, 23.835598, 23.835552, 23.835054, 23.834215, 23.833714, 23.833586, 23.828684, 23.827757, 23.825861, 23.821321, 23.819769, 23.81287, 23.805845, 23.800728, 23.794449, 23.794151, 23.791975, 23.791725, 23.788702, 23.78048, 23.778078, 23.775505, 23.767439, 23.764387, 23.757986, 23.756907, 23.7535, 23.75262, 23.744942, 23.743662, 23.74359, 23.742752, 23.742022, 23.73804, 23.724318, 23.724314, 23.722996, 23.72118, 23.71964, 23.71946, 23.70759, 23.702682, 23.701725, 23.70071, 23.700659, 23.699617, 23.698175, 23.695847, 23.693235, 23.691973, 23.69153, 23.690798, 23.689056, 23.682077, 23.68016, 23.678831, 23.674747, 23.67466, 23.673536, 23.673456, 23.672644, 23.667795, 23.650139, 23.649385, 23.646072, 23.645948, 23.644993, 23.644947, 23.634071, 23.631758, 23.62868, 23.627031, 23.626736, 23.624659, 23.616938, 23.607012, 23.607006, 23.606894, 23.606867, 23.605967, 23.60515, 23.60422, 23.600557, 23.598043, 23.594765, 23.587748, 23.58019, 23.57693, 23.576862, 23.575241, 23.574547, 23.57227, 23.567442, 23.566576, 23.565308, 23.563702, 23.5625, 23.562023, 23.558132, 23.55534, 23.550264, 23.550062, 23.548788, 23.547306, 23.546082, 23.543055, 23.540514, 23.536453, 23.5347, 23.533636, 23.53346, 23.530668, 23.528095, 23.523052, 23.520208, 23.519045, 23.518288, 23.51808, 23.515984, 23.515879, 23.515018, 23.502405, 23.502354, 23.49862, 23.498493, 23.497486, 23.49723, 23.492483, 23.491636, 23.48775, 23.485254, 23.48253, 23.481838, 23.481583, 23.48097, 23.477882, 23.47391, 23.472198, 23.471943, 23.471174, 23.471054, 23.470602, 23.470362, 23.466368, 23.46461, 23.460812, 23.45873, 23.458689, 23.458231, 23.454224, 23.452375, 23.452183, 23.450933, 23.447334, 23.442427, 23.442375, 23.439417, 23.435396, 23.435099, 23.433657, 23.43252, 23.432186, 23.43141, 23.428963, 23.425762, 23.425419, 23.41588, 23.41574, 23.412981, 23.401463, 23.401018, 23.399553, 23.397064, 23.396162, 23.394398, 23.39159, 23.390577, 23.39037, 23.388067, 23.386955, 23.38492, 23.38421, 23.379663, 23.379156, 23.361292, 23.359516, 23.358137, 23.354933, 23.352428, 23.349209, 23.349188, 23.347713, 23.346594, 23.346437, 23.344957, 23.343624, 23.343416, 23.343369, 23.342789, 23.336605, 23.332273, 23.331427, 23.329779, 23.327078, 23.325748, 23.322195, 23.321033, 23.314442, 23.31151, 23.311129, 23.30973, 23.309158, 23.308609, 23.307661, 23.299437, 23.296848, 23.294092, 23.292923, 23.292458, 23.291891, 23.291084, 23.289585, 23.286205, 23.286, 23.274527, 23.274475, 23.273153, 23.271873, 23.271511, 23.26671, 23.26668, 23.260057, 23.258715, 23.256315, 23.248419, 23.243078, 23.238205, 23.238085, 23.232174, 23.230787, 23.230228, 23.226955, 23.214281, 23.20858, 23.207012, 23.205181, 23.198732, 23.182962, 23.181091, 23.181046, 23.18016, 23.176832, 23.171648, 23.17138, 23.169456, 23.167587, 23.166769, 23.166327, 23.165115, 23.156862, 23.156693, 23.155718, 23.154964, 23.153255, 23.151262, 23.151073, 23.146484, 23.146433, 23.146126, 23.145958, 23.143448, 23.142862, 23.14081, 23.13554, 23.133486, 23.131996, 23.12851, 23.126245, 23.123817, 23.120676, 23.120533, 23.115982, 23.115866, 23.114567, 23.11371, 23.1123, 23.10985, 23.106888, 23.10597, 23.10534, 23.103104, 23.102945, 23.10136, 23.100737, 23.097725, 23.096857, 23.096794, 23.096758, 23.088463, 23.085073, 23.084509, 23.081842, 23.08177, 23.081356, 23.079506, 23.079208, 23.0783, 23.070047, 23.065971, 23.063898, 23.063723]
  out "dT_NN_Init":dbl=1.7655348999978742 format="%.2f"
  out "dT_Read_DS(Train)":dbl=0.3616576000058558 format="%.2f"
  out "dT_Read_DS(Test)":dbl=0.17860400000063237 format="%.2f"
  out "dT_Eval":dbl=1.166147700001602 format="%.2f"
  out "dT_Predict(DS)":dbl=0.1732857999886619 format="%.2f"
  out "Coreset Max":sgl=74.63289
  out "Feature Size":i32=512
  out "Coreset Min":sgl=23.063723
  in  "Online_Coreset_Params":T5={"Distance_Metric"=enum."Euclidean", "CoreSet_Size"=-1.0, "Start_idx"=3}
  out "Closest_Train_Sample":T17(plugin-control)
  in  "UpScale Factor":sgl=1.0
  in  "index":i32=24 min=0 max=24
  out "Anomaly Detection Result":T17(plugin-control)
  out "Image_Thrshld (Eval)":sgl=33.7813
  in  "Image_Thrshld(Custom)":sgl=1.0 format="%_5g"
  out "Pixel_Score(Max)":sgl=32.866966
  out "Image_File_Path":path=path "D:/Ngene/GitHub/deepltk_examples/3_Image_Processing/36_Anomaly_Detection/Dataset/Playing_Cards_3ofHearts/test/bad/(227).png"
  out "Pixel_Thrshld (Eval)":sgl=26.7008
  out "Anomaly?":bool=TRUE
  out "Img_Score":sgl=34.94818
  in  "Pixel_Thrshld(Custom)":sgl=28.1 format="%_5g"
  in  "DS Selector":enum16{"Good", "Bad", "Both"}(ring)=enum."Bad"
  in  "Order":enum16{"Ascending", "Descending", "File"}(ring)=enum."Descending"
  out "error out":errorcluster
  in  "Closest_Idx":i32 min=0 max=4
  out "#Closest_Samples":i32=5
  in  "Feature Color":u32(colorbox)=16860
  in  "ROI Scales":T18={"Receptive_Field"=1.0, "Patch"=1.0} {"Patch" min=0 max=0; "Receptive_Field" min=0 max=0}
  out "Closest_Score":sgl=22.886082
  in  "Show Patch Grid?":bool
  in  "Search Mode":bool
  in  "Heatmap Range":T16={"Min"=25.0, "Max"=32.0} {"Min" format="%#_5g"}
  in  "ROI Color":u32(colorbox)=16860
  in  "Display_Image":T19(ring)=enum."Segmentation"
  out "dT_Predict":dbl=0.005059247887094873 format="%#_3p"
  in  "Stop":bool
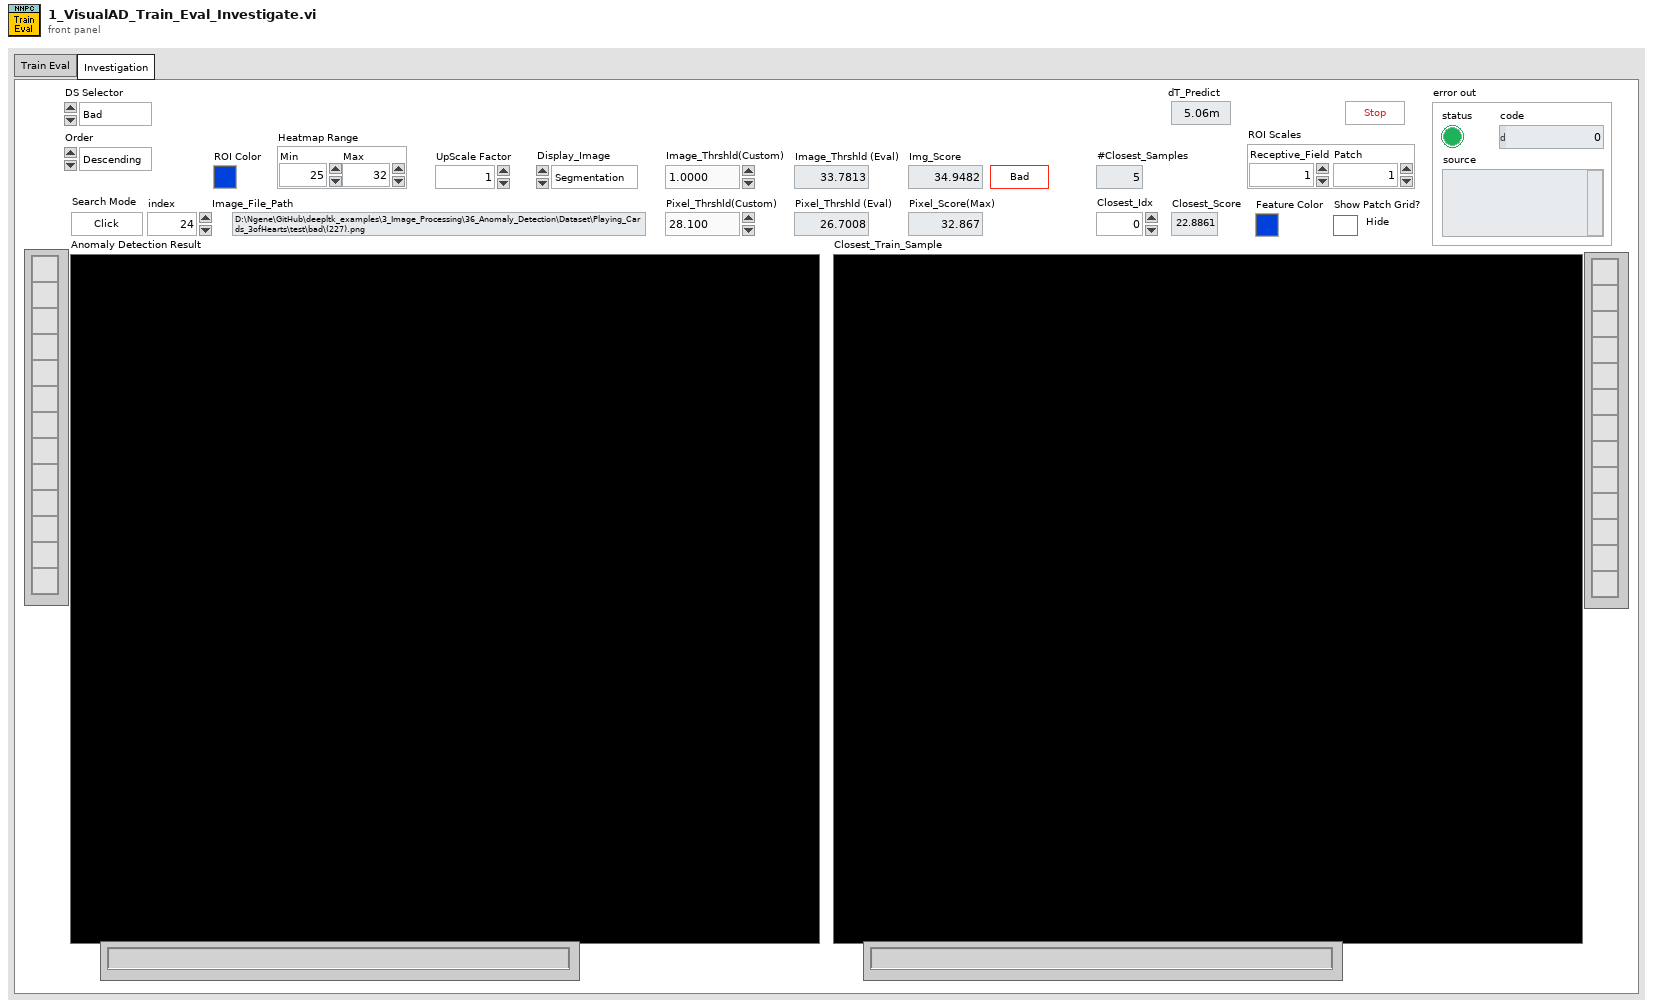
[diagram p1: front panel]
types:
  T1 = typedef "DeepLTK_Anomaly_Detection_Addon.lvlib/NN_Paths.ctl" = cluster{"CFG":path, "BIN":path}
  T2 = typedef "DeepLTK_Anomaly_Detection_Addon.lvlib/NNPC_Setup.ctl" = cluster{"Input_Dims":T3, "mBatch":i32, "Device":T4, "GPU Id":i32}
  T3 = typedef "Deep_Learning_Toolkit_by_Ngene.lvlib/NN_Dims(C,H,W).ctl" = cluster{"C":i32, "H":i32, "W":i32}
  T4 = typedef "Deep_Learning_Toolkit_by_Ngene.lvlib/NN_Device.ctl" = enum16{"CPU", "GPU"}
  T5 = typedef "DeepLTK_Anomaly_Detection_Addon.lvlib/NNPC_Coreset_Params.ctl" = cluster{"Distance_Metric":T6, "CoreSet_Size":sgl, "Start_idx":i32}
  T6 = typedef "DeepLTK_Anomaly_Detection_Addon.lvlib/Distance_Metric.ctl" = enum16{"Euclidean", "Cosine"}
  T7 = typedef "DeepLTK_Anomaly_Detection_Addon.lvlib/NNFE_CFG.ctl" = cluster{"Name":string, "Layer_Selection_By":T8, "Feature_Layers":T9, "Interpolation_Type":T10}
  T8 = typedef "DeepLTK_Anomaly_Detection_Addon.lvlib/Layer_Selector.ctl" = enum16{"Stride", "Layer_Idx"}
  T9 = typedef "DeepLTK_Anomaly_Detection_Addon.lvlib/Feature_Layer_Selector.ctl" = cluster{"[LayerID, PatchSize]":cluster{"Layer_ID":i32, "Patch_Size":i32}[]}
  T10 = typedef "DeepLTK_Anomaly_Detection_Addon.lvlib/Interpolation_Selector.ctl" = enum16{"Nearest", "Bi-Linear"}
  T11 = typedef "DeepLTK_Anomaly_Detection_Addon.lvlib/NNPC_Random_Projection_CFG.ctl" = cluster{"Method":T12, "Target_Dim":i32, "Seed":i32}
  T12 = typedef "DeepLTK_Anomaly_Detection_Addon.lvlib/Dim_Reduction_Method.ctl" = enum16{"None", "Rnd_Proj", "PCA"}
  T13 = typedef "DeepLTK_Anomaly_Detection_Addon.lvlib/Evaluation_Metrics(Pixel_Image).ctl" = cluster{"Evaluation_Metrics(Pixel)":T14, "Evaluation_Metrics(Image)":T14}
  T14 = typedef "DeepLTK_Anomaly_Detection_Addon.lvlib/Evaluation_Metrics.ctl" = cluster{"Scores(Good)":cluster{"X Values":dbl[], "Histogram: h(x)":i32[]}, "Scores(Bad)":cluster{"X Values":dbl[], "Histogram: h(x)":i32[]}, "Eval Stats":T15}
  T15 = typedef "DeepLTK_Anomaly_Detection_Addon.lvlib/Eval_Results.ctl" = cluster{"Scores(Good)":T16, "Scores(Bad)":T16, "# of Samples(Good)":i32, "# of Samples(Bad)":i32, "AUROC":sgl, "F1_Max":sgl, "Thrshld(F1_Max)":sgl, "Prec.(F1_Max)":sgl, "Recall(F1_Max)":sgl, "FPR(F1_Max)":sgl, "FNR(F1_Max)":sgl}
  T16 = typedef "DeepLTK_Anomaly_Detection_Addon.lvlib/MinMax.ctl" = cluster{"Min":sgl, "Max":sgl}
  T17 = typedef "IMAQ Image.ctl" = refnum<image>
  T18 = typedef "Patch_RF_Scales.ctl" = cluster{"Receptive_Field":sgl, "Patch":sgl}
  T19 = enum16{"Original", "Ground_Truth", "HeatMap", "Mask", "Segmentation"}
  T20 = typedef "DeepLTK_Anomaly_Detection_Addon.lvlib/Crop_CFG.ctl" = cluster{"Left":sgl, "Top":sgl, "Right":sgl, "Bottom":sgl}
  T21 = typedef "Image Type" = u32
  T22 = typedef "DeepLTK_Anomaly_Detection_Addon.lvlib/Feature_Scorer_Params.ctl" = cluster{"Nearest_Neighbors":i32, "Calculate Anomaly Map":bool, "Gaussian_Blur":T23}
  T23 = typedef "DeepLTK_Anomaly_Detection_Addon.lvlib/Gaussian_Blur.ctl" = cluster{"Kernel_Size":i32, "Sigma":sgl}
  T24 = typedef "Detection_Results.ctl" = cluster{"Image Score":sgl, "Pixel Score":sgl[][], "File Path":path}
  T25 = typedef "Read_Options.ctl" = cluster{"Read Bads?":bool, "Read GTs?":bool, "Update. DS Stats?":bool}
  T26 = typedef "DeepLTK_Anomaly_Detection_Addon.lvlib/NNPC_PreProcessing_Options.ctl" = cluster{"DS_Name":string, "Input_Dims":T3, "Cropping":T20, "Interpolation Type":u32, "MultiStage_ReSample?":bool, "Dataset_Stats":T27}
  T27 = typedef "DeepLTK_Anomaly_Detection_Addon.lvlib/NNPC_DS_Stats.ctl" = cluster{"means":T28, "stds":T28}
  T28 = typedef "DeepLTK_Anomaly_Detection_Addon.lvlib/Image_Stats_RGB.ctl" = cluster{"R":sgl, "G":sgl, "B":sgl}
  T29 = typedef "Deep_Learning_Toolkit_by_Ngene.lvlib/NN_DataSet(In3D_Out3D).ctl" = cluster{"Dataset_Size":i32, "Dims_In":T3, "Labels":string[], "File Paths":path[], "Outputs Ref.":T30, "Inputs Ref.":variant, "Dims_Out":T3, "Custom_Data":variant}
  T30 = typedef "Deep_Learning_Toolkit_by_Ngene.lvlib/NN_Data_ref(4D_SGL).ctl" = refnum<data-value>
  T31 = typedef "DeepLTK_Anomaly_Detection_Addon.lvlib/NNPC_Instance.ctl" = cluster{"Name":string, "NN":T32, "MemBank_Data":T46}
  T32 = typedef "Deep_Learning_Toolkit_by_Ngene.lvlib/NN.ctl" = cluster{"Name":string, "No of Layers":i32, "mBatch":i32, "Layers":T33[], "Dimty":T34, "Dims_In":T3, "Dims_Out":T3, "Working_Dir":path, "Train?":bool, "Train_Params":T35, "LR_Update_Policy":T38, "Session Data":T40, "Ground_truth":T41, "NNg_hdls":T42, "NN_Device":T4, "GPU Id":i32, "Labels":string[], "Loss_Type":T43, "Loss_Cfg_Prms":variant, "NNG_WS":T44, "DryRun?":bool}
  T33 = typedef "Deep_Learning_Toolkit_by_Ngene.lvlib/NN_Layer_ref.ctl" = refnum<file>
  T34 = typedef "Deep_Learning_Toolkit_by_Ngene.lvlib/NN_In_Out_Dim-ty.ctl" = enum8{"In1D_Out1D", "In3D_Out1D", "In3D_Out3D", "In3D_OutBBox"}
  T35 = typedef "Deep_Learning_Toolkit_by_Ngene.lvlib/NN_Train_Params.ctl" = cluster{"Optimizer":T36, "Beta_1":sgl, "Beta_2":sgl, "Weight Decay(L1)":sgl, "Weight Decay(L2)":sgl, "Data_Sampling":T37}
  T36 = typedef "Deep_Learning_Toolkit_by_Ngene.lvlib/NN_Train_Optimizer.ctl" = enum16{"SGD", "Adam", "Adagrad", "Adadelta", "RMSProp", "Nesterov"}
  T37 = typedef "Deep_Learning_Toolkit_by_Ngene.lvlib/NN_Train_Data_Sampling.ctl" = enum16{"Random", "Sequential"}
  T38 = typedef "Deep_Learning_Toolkit_by_Ngene.lvlib/NN_LR_Policy_Cfg.ctl" = cluster{"Policy_Type":T39, "LR0":dbl, "k":sgl, "WarmUp_Policy":enum16{"Step", "Ramp"}, "WarmUp_Iter":i32, "WarmUp_Ratio":sgl}
  T39 = typedef "Deep_Learning_Toolkit_by_Ngene.lvlib/NN_LR_Policy_Type.ctl" = enum16{"Manual", "Step", "Exp", "1/t"}
  T40 = typedef "Deep_Learning_Toolkit_by_Ngene.lvlib/NN_Train_Session_Data.ctl" = cluster{"Epochs":sgl, "Tot_Iter":i32, "LR":sgl, "LR_iter":i32}
  T41 = typedef "Deep_Learning_Toolkit_by_Ngene.lvlib/NN_Ground_truth.ctl" = cluster{"Y":variant}
  T42 = typedef "Deep_Learning_Toolkit_by_Ngene.lvlib/nng_cuda_handles.ctl" = cluster{"cudnn":u64, "cublas":u64, "stream":u64, "curand":u64}
  T43 = typedef "Deep_Learning_Toolkit_by_Ngene.lvlib/NN_Loss_Type.ctl" = enum16{"None", "MSE", "CrossEntropy", "YOLO_v2", "YOLO_v4"}
  T44 = typedef "Deep_Learning_Toolkit_by_Ngene.lvlib/NNG_WS.ctl" = cluster{"NNG_WS_Mem":T45, "Max_WS_Size":i64}
  T45 = typedef "Deep_Learning_Toolkit_by_Ngene.lvlib/NNg_WS_Mem_DVR.ctl" = refnum<data-value>
  T46 = typedef "DeepLTK_Anomaly_Detection_Addon.lvlib/MemBank_and_Norm_Variants.ctl" = cluster{"MemBank":variant, "MemBank Norm":variant}
  T47 = typedef "DeepLTK_Anomaly_Detection_Addon.lvlib/Feature_Coords(Idx,i,j).ctl" = cluster{"Idx":i32, "i":i32, "j":i32}
  T48 = typedef "imagedata.ctl" = cluster{"image type":i32, "image depth":i32, "image":u8[], "mask":u8[], "colors":u32[], "Rectangle":cluster{"left":i16, "top":i16, "right":i16, "bottom":i16}}
  T49 = typedef "DeepLTK_Anomaly_Detection_Addon.lvlib/NNPC_Evaluation_Results.ctl" = cluster{"Threshold(Image)":sgl, "Threshold(Pixel)":sgl, "Pixel_Range":cluster{"Min":sgl, "Max":sgl}}
  T50 = typedef "Selected_Coreset_Elements_and_Dim_Stride_Info.ctl" = cluster{"Dims_Out":T51, "Stride":i32, "Coreset_Elements":T47[]}
  T51 = typedef "Dims(2D)ctl.ctl" = cluster{"H":i32, "W":i32}
  T52 = typedef "Deep_Learning_Toolkit_by_Ngene.lvlib/NN_Layer.ctl" = cluster{"Name":string, "Layer_Data":T53, "Layer_Type":T54, "Dims_In":T3, "Layers_In":T33[], "Dims_Out":T3, "Layers_Out":T33[], "Metrics":T55, "GPU_Data":T56, "mBatch":i32, "NN_Device":T4, "NNg_hdls":T42, "Train?":bool, "Dimty":T57, "RecptField":T58, "Idx":i32}
  T53 = typedef "Deep_Learning_Toolkit_by_Ngene.lvlib/NN_Layer_Data_Refnum.ctl" = refnum<file>
  T54 = typedef "Deep_Learning_Toolkit_by_Ngene.lvlib/NN_Layer_Type.ctl" = enum16{"Input1D", "Input3D", "Conv1D", "Conv2D", "Conv2D_Adv", "MaxPool", "AvgPool", "UpSample", "DropOut3D", "ShortCut", "Concat", "SoftMax3D", "FC", "DropOut", "Softmax", "Flatten", "YOLO_v2", "YOLO_v4", "Activation", "BatchNormalization", "LayerNormalization", "Scale", "Unsupported"}
  T55 = typedef "Deep_Learning_Toolkit_by_Ngene.lvlib/NN_Layer_Metrics.ctl" = cluster{"Data":dbl, "Params":dbl, "Ops":dbl}
  T56 = typedef "Deep_Learning_Toolkit_by_Ngene.lvlib/NNg_Layer_Data_Refnum.ctl" = refnum<file>
  T57 = typedef "Deep_Learning_Toolkit_by_Ngene.lvlib/NN_Layer_Dimty.ctl" = enum16{"1D", "3D"}
  T58 = typedef "Deep_Learning_Toolkit_by_Ngene.lvlib/NN_Layer_RF_State.ctl" = cluster{"Dims":T59, "J":T59}
  T59 = typedef "Deep_Learning_Toolkit_by_Ngene.lvlib/NN_Dims(V,H).ctl" = cluster{"V":i32, "H":i32}
  T60 = typedef "Display_Options.ctl" = cluster{"ROI_Options":T61, "Heatmap_Options":T62, "Report_Images_CFG":T64}
  T61 = typedef "ROI_Display_Options.ctl" = cluster{"Color":u32, "Width":u32, "Drawing Mode":enum16{"Frame", "Fill"}}
  T62 = typedef "Heatmap_Display_Options.ctl" = cluster{"ColorMap":T63, "Alpha":sgl, "Heatmap Range":T16}
  T63 = typedef "ColorMap.ctl" = enum16{"Jet", "Perula", "Inferno", "Plasma", "Viridis"}
  T64 = typedef "Report_Images_CFG.ctl" = cluster{"Original Image":bool, "Ground Truth":bool, "HeatMap":bool, "Mask":bool, "Segmentation":bool}
  T65 = typedef "Anomaly_Detection_Results_Imgs.ctl" = cluster{"Image":T17, "Ground Truth":T17, "Predicted Heat Map":T17, "Predicted Mask":T17, "Segmentation":T17}
  T66 = typedef "Closest_Sample_Info.ctl" = cluster{"Score":sgl, "Feature_Coords":T47}
  T67 = typedef "Deep_Learning_Toolkit_by_Ngene.lvlib/NN_BBox.ctl" = cluster{"x":sgl, "y":sgl, "w":sgl, "h":sgl}
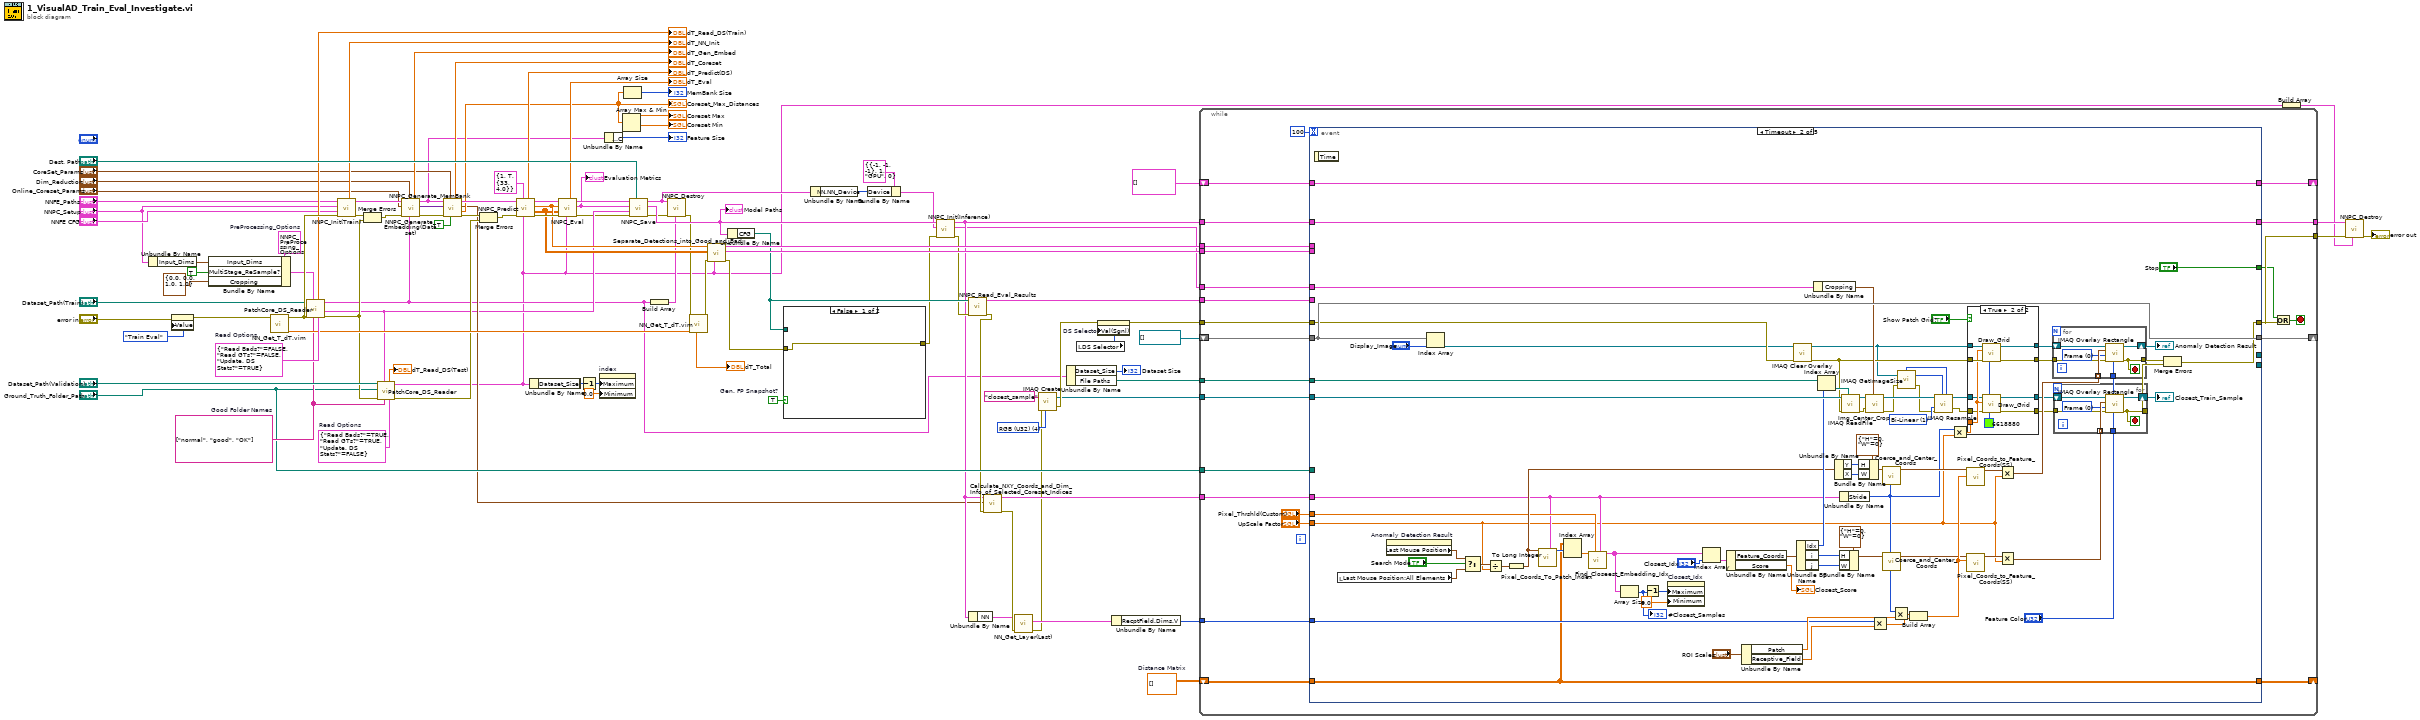
[diagram p0: block diagram]
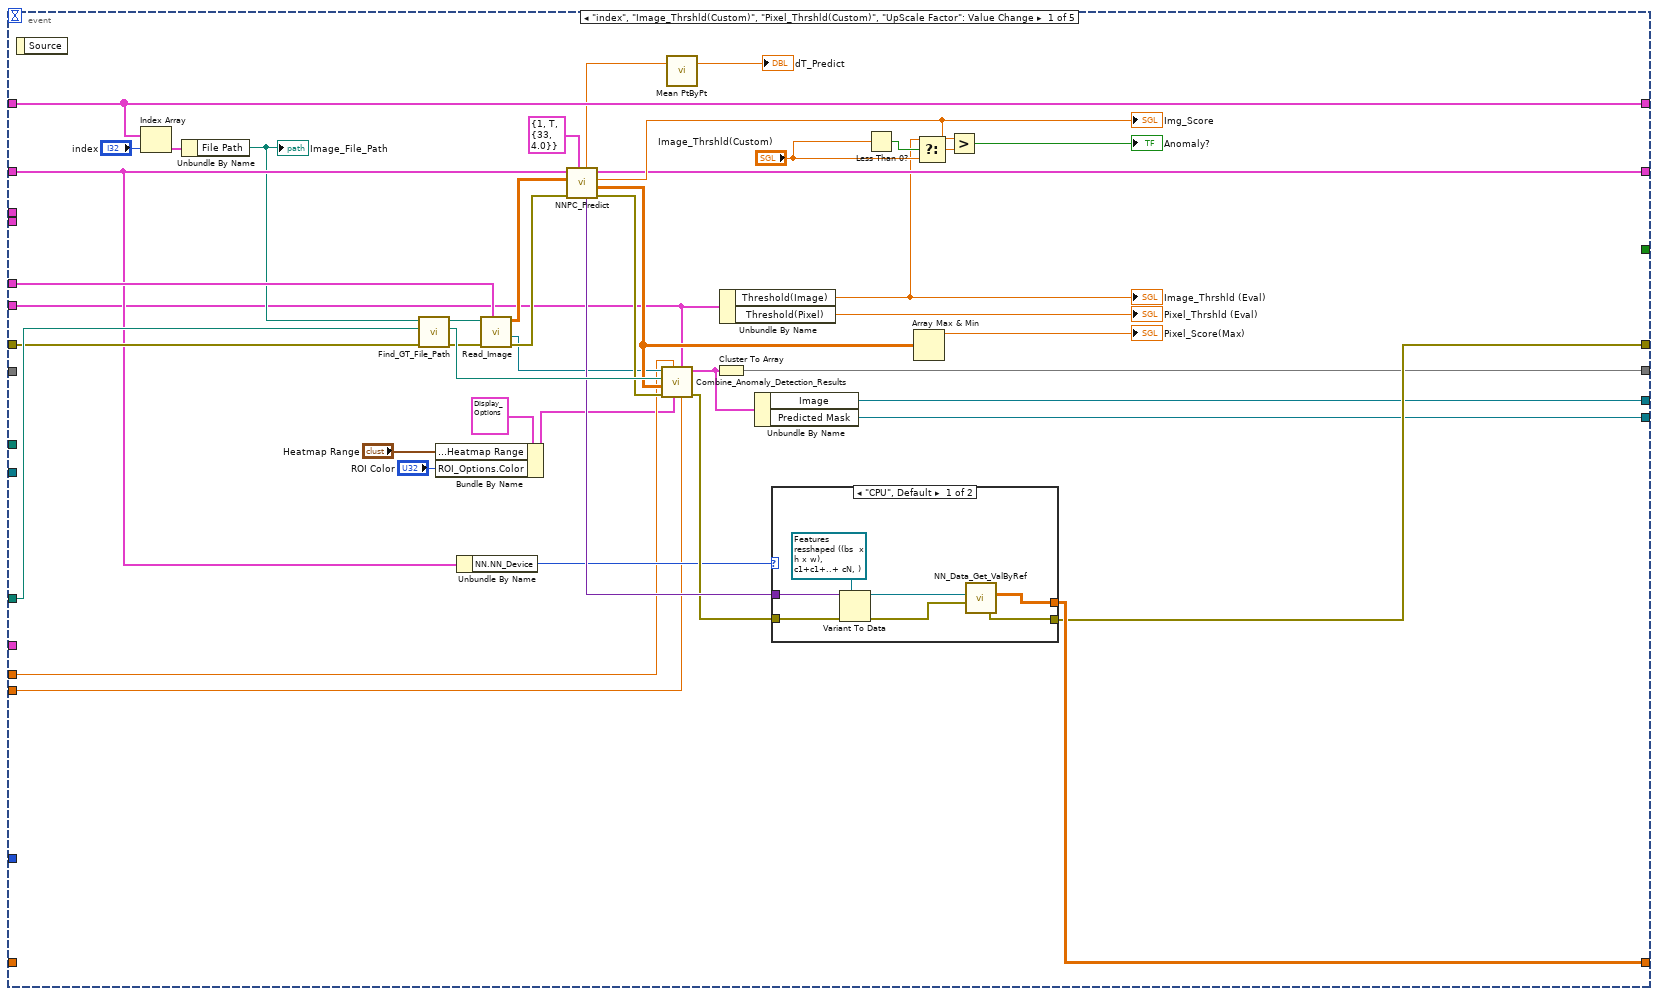
[diagram p2: hidden frame]
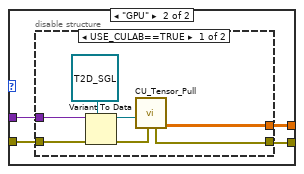
[diagram p3: hidden frame]
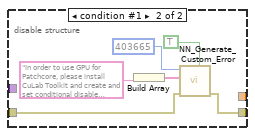
[diagram p4: hidden frame]
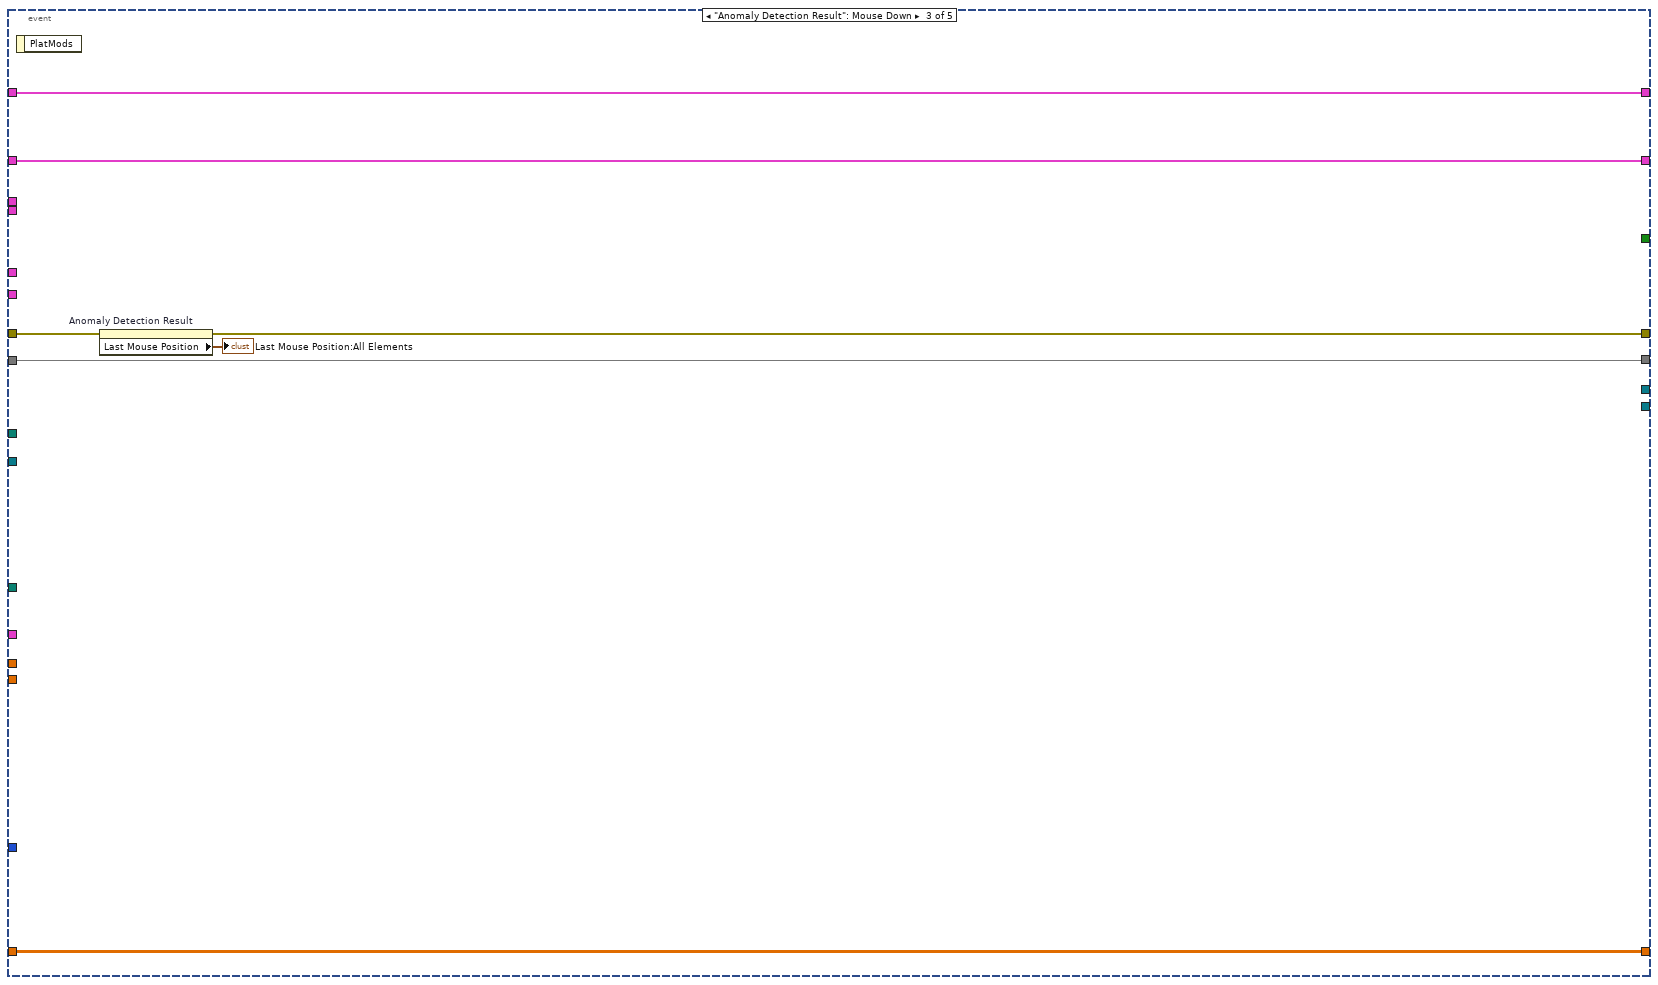
[diagram p6: hidden frame]
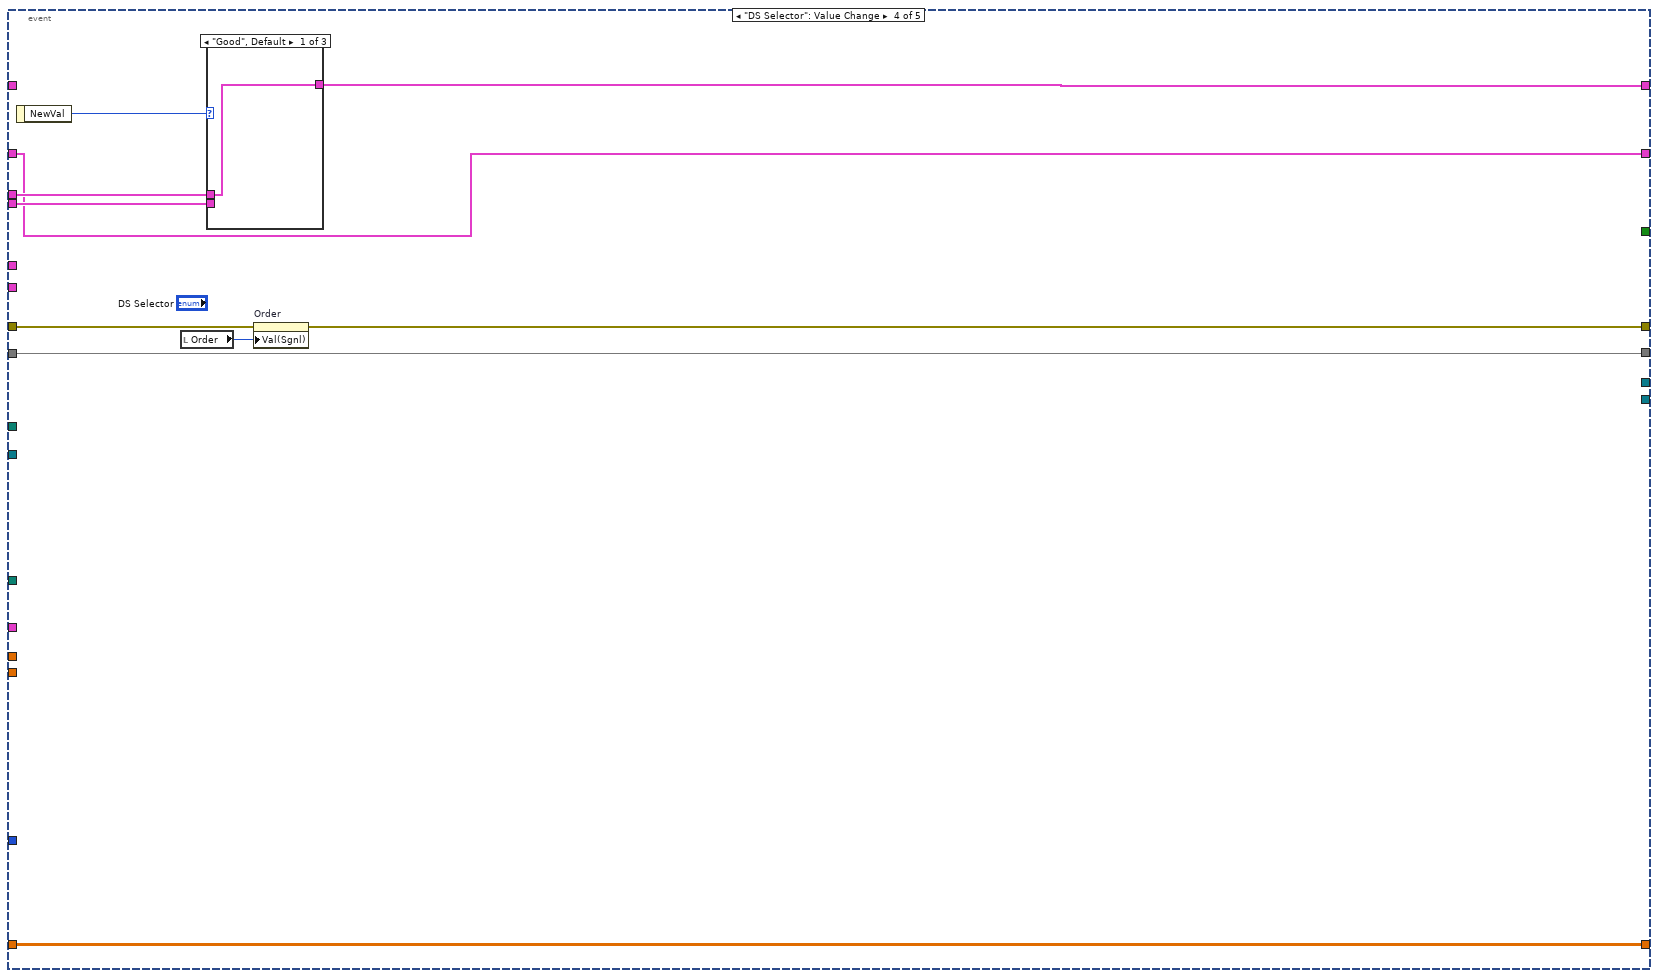
[diagram p7: hidden frame]
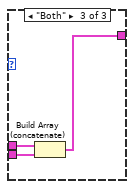
[diagram p9: hidden frame]
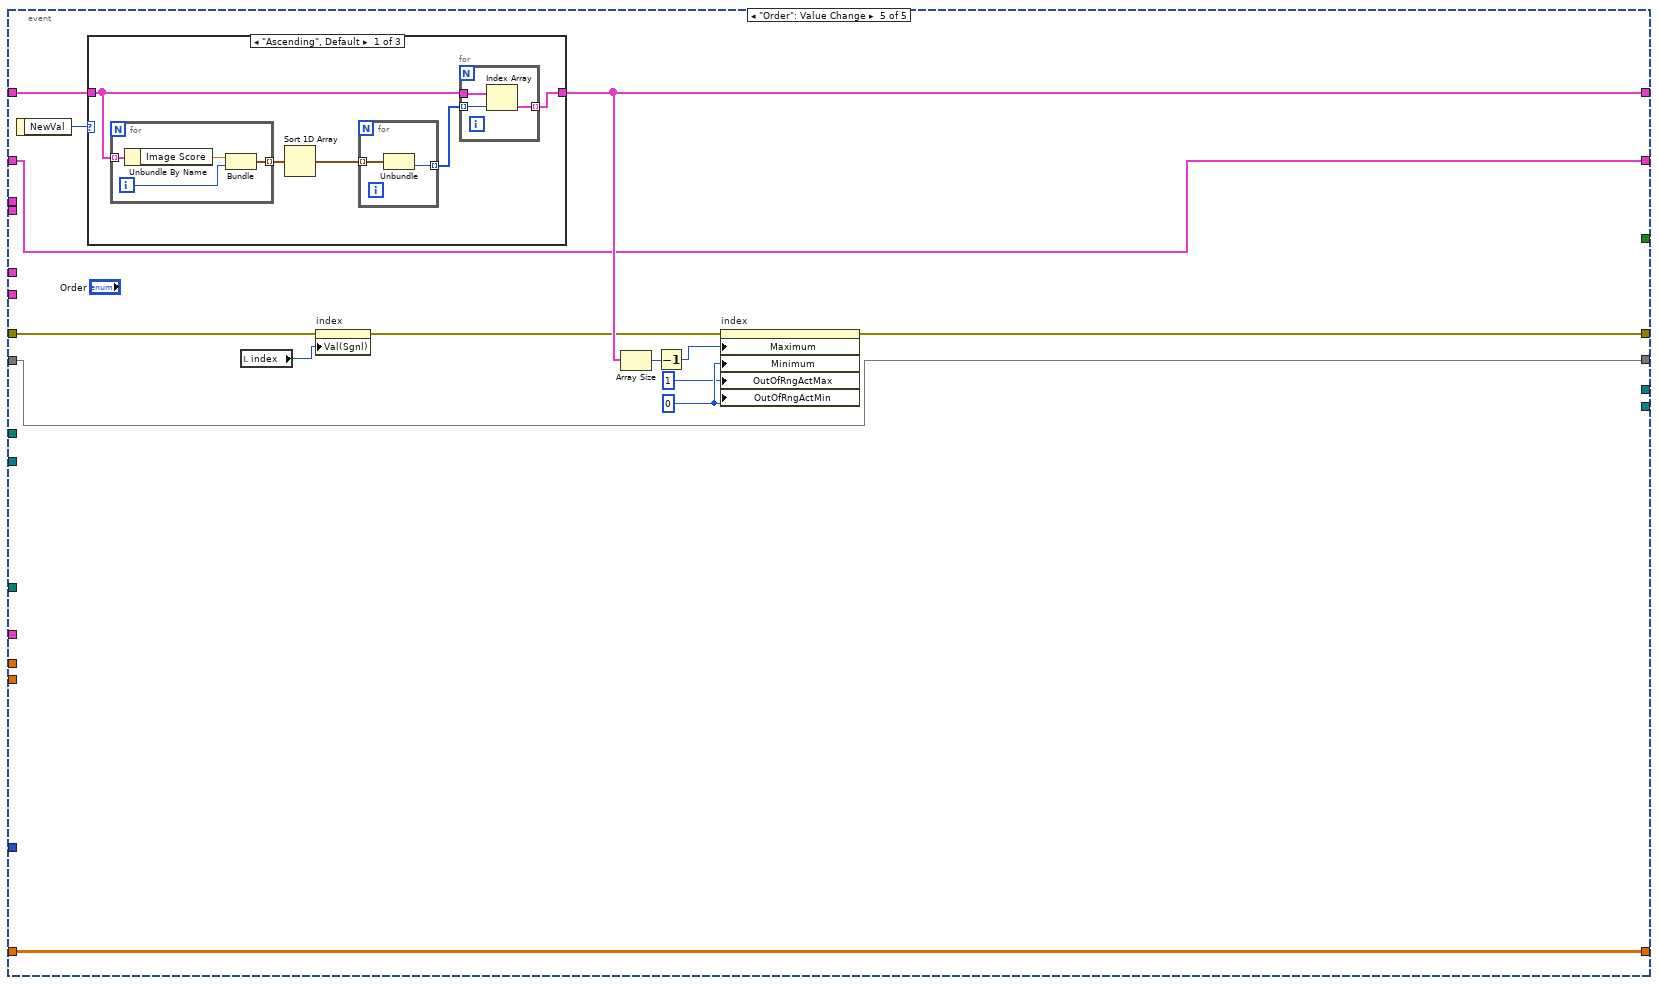
[diagram p10: hidden frame]
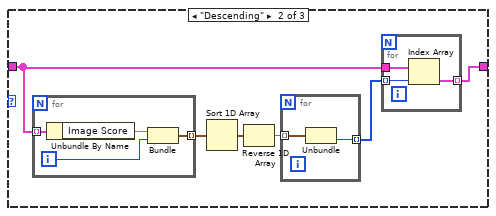
[diagram p11: hidden frame]
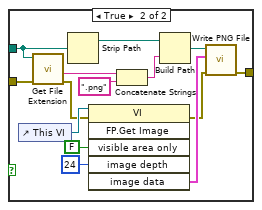
[diagram p13: hidden frame]
diagram:
  w37 = T21 4 items=["Grayscale (U8)", "Grayscale (I16)", "Grayscale (SGL)", "Complex (CSG)", "RGB (U32)", "HSL (U32)", "RGB (U64)", "Grayscale (U16)"] ("Image Type")
  w38 = sgl[][] []  # Distance Matrix
  w69 = TRUE  # Gen. FP Snapshot?
  w85 = T25 {"Read Bads?"=TRUE, "Read GTs?"=TRUE, "Update. DS Stats?"=FALSE}  # Read Options
  w96 = T26 {"DS_Name"="", "Input_Dims"={"C"=3, "H"=224, "W"=224}, "Cropping"={"Left"=0.0, "Top"=1.0, "Right"=0.0, "Bottom"=1.0}, "Interpolation Type"=1, "MultiStage_ReSample?"=FALSE, "Dataset_Stats"={"means"={"R"=0.0, "G"=0.0, "B"=0.0}, "stds"={"R"=1.0, "G"=1.0, "B"=1.0}}}  # PreProcessing_Options
  w93 = T25 {"Read Bads?"=FALSE, "Read GTs?"=FALSE, "Update. DS Stats?"=TRUE}  # Read Options
  w75 = string[] ["normal", "good", "OK"]  # Good Folder Names
  n1 = Unbundle By Name("NNPC_Setup") -> ("Input_Dims"=w94:T3)
  n2 = property class="TabCtl (strict)"(error in="error in", "Value"=enum32{"Train Eval", "Investigation"}."Train Eval") -> (error out=w61:errorcluster)  [unwired: 1 in, 1 out]
  n3 = Bundle By Name(cluster=w96, "Input_Dims"=w94, "MultiStage_ReSample?"=TRUE ("Multi-Stage_DownSample?"), "Cropping"=T20 {"Left"=0.0, "Top"=0.0, "Right"=1.0, "Bottom"=1.0} ("Crop_CFG")) -> (w53:T26)
  n4 = call "NN_Get_T_dT.vim"("error in"=w61) -> ("T_out"=w90:dbl, "error out"=w104:errorcluster)  [unwired: 6 in, 1 out]
  n5 = call "PatchCore_DS_Reader.vi"("Read Options"=w93, "Good Unique Labels"=w75, "PreProc_Options_in"=w53, "error in"=w104, "Folder Path"="Dataset_Path(Train)") -> ("error out"=w82:errorcluster, "PreProc_Options_out"=w13:T26, "Dataset"=w3:T29, "dT_DS_Reader"=→"dT_Read_DS(Train)":dbl)  [unwired: 3 in]
  n6 = call <vilib>:"NNPC_Init(Train).vi"("error in"=w104, "NNFE_CFG"="NNFE CFG", "NNPC_Setup"="NNPC_Setup", "NNFE_Paths"="NNFE_Paths") -> ("error out"=w100:errorcluster, "NNPC_out"=w99:T31, "dT_Init_Train"=→"dT_NN_Init":dbl)  [unwired: 5 in]
  n7 = Merge Errors(w100, w82) -> (w91:errorcluster)
  n8 = call "PatchCore_DS_Reader.vi"("Read Options"=w85, "Good Unique Labels"=w75, "PreProc_Options_in"=w13, "error in"=w82, "GT Folder Path"="Ground_Truth_Folder_Path", "Folder Path"="Dataset_Path(Validation)") -> ("error out"=w76:errorcluster, "Dataset"=w2:T29, "dT_DS_Reader"=→"dT_Read_DS(Test)":dbl)  [unwired: 2 in, 1 out]
  n9 = call <vilib>:"NNPC_Generate_Embedding(Dataset).vi"("Dataset"=w3, "Dim_Reduction"="Dim_Reduction", "error in"=w91, "Online_Coreset_Params"="Online_Coreset_Params", "NNPC_in"=w99) -> ("error out"=w29:errorcluster, "Feature_Embeddings"=w87:variant, "NNPC_out"=w54:T31, "dT_Embed"=→"dT_Gen_Embed":dbl)  [unwired: 2 in, 1 out]
  n10 = call <vilib>:"NNPC_Generate_MemBank.vi"("Destroy Embeds Afterwards?"=TRUE, "Coreset_Params"="CoreSet_Params", "error in"=w29, "Feature_Embeddings"=w87, "NNPC_in"=w54) -> ("error out"=w70:errorcluster, "Max_Distances"=w56:sgl[], "Selected_Feature_Coords"=w17:T47[], "NNPC_out"=w78:T31, "dT_Coreset"=→"dT_Coreset":dbl)  [unwired: 2 in]
  "Coreset_Max_Distances" <- w56
  n11 = Merge Errors(w70, w76) -> (w77:errorcluster)
  n12 = call-poly <vilib>:"NNPC_Predict.vi"("Dataset"=w2, "Feature_Scorer_Params"=T22 {"Nearest_Neighbors"=1, "Calculate Anomaly Map"=TRUE, "Gaussian_Blur"={"Kernel_Size"=33, "Sigma"=4.0}}, "error in"=w77, "NNPC_in"=w78) -> ("error out"=w79:errorcluster, "Anomaly_Maps"=w66:sgl[][][], "Pred_Scores"=w67:sgl[], "NNPC_out"=w74:T31, "dT_Predict"=→"dT_Predict(DS)":dbl)  [unwired: 3 in]
  n13 = Unbundle By Name(w2) -> ("Dataset_Size"=w47:i32)
  n14 = call <vilib>:"NNPC_Eval.vi"("Dataset"=w2, "error in"=w79, "Anomaly_Maps"=w66, "Pred_Scores"=w67, "NNPC_in"=w74) -> ("error out"=w9:errorcluster, "Evaluation_Metrics"=w4:T13, "NNPC_out"=w73:T31, "dT_Eval"=→"dT_Eval":dbl)  [unwired: 3 in]
  "Evaluation Metrics" <- w4
  n15 = Decrement(x=w47) -> (x-1=w49:i32)
  n16 = property on="index" class="DigNum (strict)"("Maximum"=w49, "Minimum"=0.0 ("Data Entry Limits:Minimum")) -> ()  [unwired: 2 in, 2 out]
  n17 = Unbundle By Name(w54) -> ("NN.Dims_Out.C"=→"Feature Size":i32)
  n18 = Array Max & Min(array=w56) -> (max value=→"Coreset Max":sgl, min value=→"Coreset Min":sgl)  [unwired: 2 out]
  n19 = Array Size(array=w56) -> (size(s)=→"MemBank Size":i32)
  n20 = call <vilib>:"NNPC_Save.vi"("Dst_Folder"="Dest. Path", "error in"=w9, "PreProc_Options_in"=w13, "Evaluation Metrics"=w4, "NNPC_in"=w73) -> ("error out"=w11:errorcluster, "NNPC_Paths"=w50:T1, "NNPC_out"=w42:T31)  [unwired: 4 in]
  "Model Paths" <- w50
  n21 = Build Array(w3) -> (w5:T29[])
  n22 = call <vilib>:"NNPC_Destroy.vi"("Datasets_to_Destroy"=w5, "error in"=w11, "NNPC_in"=w42) -> ("error out"=w8:errorcluster)  [unwired: 8 in]
  n23 = call "NN_Get_T_dT.vim"("T_in"=w90, "error in"=w8) -> ("error out"=w7:errorcluster, "dT"=→"dT_Total":dbl)  [unwired: 5 in, 1 out]
  n24 = call "Separate_Detections_into_Good_and_Bad.vi"("Dataset"=w2, "error in"=w7, "Pixel Scores"=w66, "Image Scores"=w67) -> ("error out"=w6:errorcluster, "Bad Samples"=w63:T24[], "Good Samples"=w62:T24[])  [unwired: 5 in]
  n25 = Unbundle By Name(w50) -> ("CFG"=w52:path)
  n26 = case shown="False" w69 {
    tunnel: w52 -> [_ w109]
    tunnel: [w105 w108] -> w32
    tunnel: w6 -> [w105 w107]
    frame False {
    }
    frame True {
      n27 = control-ref of="This VI"() -> (w119:refnum<vi>)
      n28 = call <vilib>:"Get File Extension.vi"("error in (no error)"=w107, "file"=w109) -> ("error out"=w106:errorcluster, "filename without extension"=w114:string)  [unwired: 5 in, 3 out]
      n29 = Strip Path(path=w109) -> (stripped path=w111:path)  [unwired: 1 out]
      n30 = invoke class="VI" method="FP.Get Image"(reference=w119, error in=w106, "visible area only"=FALSE ("Visible Area Only"), "image depth"=24 ("Image Depth")) -> (error out=w115:errorcluster, "image data"=w116:T48)  [unwired: 2 in, 4 out]
      n31 = Concatenate Strings(w114, ".png" ("string")) -> (w112:string)
      n32 = Build Path(base path=w111, name or relative path=w112) -> (appended path=w110:path)
      n33 = call <vilib>:"Write PNG File.vi"("error in (no error)"=w115, "image data"=w116, "path to PNG file"=w110) -> ("error out"=w108:errorcluster)  [unwired: 7 in, 1 out]
    }
  }
  n34 = Unbundle By Name(w42) -> ("NN.NN_Device"=w40:T4)
  n35 = Bundle By Name(cluster=T2 {"Input_Dims"={"C"=-1, "H"=-1, "W"=-1}, "mBatch"=1, "Device"=enum."GPU", "GPU Id"=0} ("NNPC_Setup"), "Device"=w40) -> (w41:T2)
  n36 = call <vilib>:"NNPC_Init(Inference).vi"("error in"=w32, "NNPC_Setup"=w41, "NNPC_Paths"=w50) -> ("error out"=w31:errorcluster, "PreProc_Options"=w12:T26, "NNPC_out"=w23:T31)  [unwired: 4 in, 2 out]
  n37 = call <vilib>:"NNPC_Read_Eval_Results.vi"("error in (no error)"=w31, "CFG file path"=w52) -> ("error out"=w24:errorcluster, "Evaluation_Results"=w51:T49)  [unwired: 8 in]
  n38 = Unbundle By Name(w23) -> ("NN"=w21:T32)
  n39 = call "Calculate_NXY_Coords_and_Dim_Info_of_Selected_Coreset_Indices.vi"("error in (no error)"=w24, "Selected_Feature_Coords"=w17, "NNPC_Instance"=w23) -> ("error out"=w25:errorcluster, "Selected_Coreset_Element_Info"=w26:T50)  [unwired: 7 in]
  n40 = call <vilib>:"NN_Get_Layer(Last).vi"("error in (no error)"=w25, "NN in"=w21) -> ("error out"=w22:errorcluster, "Last_Layer"=w28:T52)  [unwired: 6 in, 2 out]
  n41 = call "IMAQ Create"("Image Name"="closest_sample", "Image Type"=w37, "error in (no error)"=w22) -> ("New Image"=w34:T17, "error out"=w35:errorcluster)  [unwired: 2 in]
  n42 = Unbundle By Name(w3) -> ("Dataset_Size"=→"Dataset Size":i32, "File Paths"=w19:path[])
  n43 = local read "DS Selector"() -> (w64:enum16{"Good", "Bad", "Both"})
  n44 = property on="DS Selector" class="Enum (strict)"(error in=w35, "Val(Sgnl)"=w64) -> (error out=w44:errorcluster)  [unwired: 1 in, 1 out]
  n45 = Unbundle By Name(w28) -> ("RecptField.Dims.V"=w27:i32)
  n46 = while {
    tunnel: "Ground_Truth_Folder_Path" -> [w142]
    tunnel: w62 -> [w141]
    tunnel: w63 -> [w140]
    shift-right: [w139] -> _
    shift-left: T24[] [] ("Bad Samples") -> [w138]
    tunnel: w12 -> [w136]
    tunnel: w51 -> [w135]
    tunnel: w23 -> [w134]
    tunnel: w27 -> [w133]
    tunnel: w26 -> [w132]
    tunnel: w19 -> [w131]
    tunnel: [w130] -> w20
    shift-right: [w129] -> _
    shift-left: w38 -> [w128]
    shift-right: [w125] -> _
    shift-left: T17[] [] ("Anomaly Detection Rresults") -> [w124]
    tunnel: w34 -> [w122]
    tunnel: w44 -> [w143]
    tunnel: [w127] -> w18
    stop <- w137 stop-if-true
    n47 = event shown="[1] Timeout" {
      selector: _ -> [_ _ _ _ _]
      dyn-events: _ -> [_ _ _ _ _]
      timeout: 100 -> [_ _ _ _ _]
      tunnel: w143 -> [w181 w265 w324 w330 w346]
      tunnel: [w162 w231 w323 w329 w344] -> w127
      tunnel: w142 -> [w182 _ _ _ _]
      tunnel: w141 -> [_ _ _ w334 _]
      tunnel: w140 -> [_ _ _ w333 _]
      tunnel: [w168 w290 w321 w332 w351] -> w139
      tunnel: w138 -> [w168 w290 w321 _ w353]
      tunnel: w136 -> [w169 w220 _ _ _]
      tunnel: w135 -> [w150 _ _ _ _]
      tunnel: w134 -> [w163 w289 w319 w326 w342]
      tunnel: w133 -> [_ w271 _ _ _]
      tunnel: w132 -> [_ w240 _ _ _]
      tunnel: w131 -> [_ w270 _ _ _]
      tunnel: [w165 w289 w319 w326 w342] -> w130
      tunnel: [w164 w268 w322 w328 w343] -> w129
      tunnel: w128 -> [_ w268 w322 w328 w343]
      tunnel: w124 -> [_ w267 w320 w327 w341]
      tunnel: [_ "Stop" _ _ _] -> w126
      tunnel: [w147 w267 w320 w327 w341] -> w125
      tunnel: w122 -> [_ w266 _ _ _]
      tunnel: "UpScale Factor" -> [w156 w222 _ _ _]
      tunnel: "Pixel_Thrshld(Custom)" -> [w155 w241 _ _ _]
      tunnel: [w144 _ _ _ _] -> _
      tunnel: [w145 _ _ _ _] -> _
      event "index", "Image_Thrshld(Custom)", "Pixel_Thrshld(Custom)", "UpScale Factor": Value Change {
        n48 = event-data() -> ()  [unwired: 1 in, 1 out]
        n49 = Index Array(array=w168, index="index") -> (element=w180:T24)
        n50 = Unbundle By Name(w180) -> ("File Path"=w159:path)
        "Image_File_Path" <- w159
        n51 = call "Find_GT_File_Path.vi"("error in"=w181, "GT Mask Folder Path"=w182, "Image File Path"=w159) -> ("error out"=w177:errorcluster, "GT File Path"=w185:path, "Image File Path out"=w178:path)  [unwired: 5 in, 1 out]
        n52 = Bundle By Name(cluster=T60 {"ROI_Options"={"Color"=16717824, "Width"=3, "Drawing Mode"=enum."Frame"}, "Heatmap_Options"={"ColorMap"=enum."Jet", "Alpha"=0.4, "Heatmap Range"={"Min"=0.089999996, "Max"=0.18}}, "Report_Images_CFG"={"Original Image"=TRUE, "Ground Truth"=TRUE, "HeatMap"=TRUE, "Mask"=TRUE, "Segmentation"=TRUE}} ("Display_Options"), "Heatmap_Options.Heatmap Range"="Heatmap Range", "ROI_Options.Color"="ROI Color") -> (w153:T60)
        n53 = Unbundle By Name(w163) -> ("NN.NN_Device"=w166:T4)
        n54 = call "Read_Image.vi"("PreProcessing_Options"=w169, "error in"=w177, "Img Path"=w178) -> ("error out"=w175:errorcluster, "Image Out(Cropped)"=w157:T17, "Image Out (Preproc)"=w158:sgl[][][])  [unwired: 3 in, 3 out]
        n55 = call-poly <vilib>:"NNPC_Predict.vi"("Feature_Scorer_Params"=T22 {"Nearest_Neighbors"=1, "Calculate Anomaly Map"=TRUE, "Gaussian_Blur"={"Kernel_Size"=33, "Sigma"=4.0}}, "error in"=w175, "Image_in"=w158, "NNPC_in"=w163) -> ("error out"=w171:errorcluster, "Anomaly_Map"=w173:sgl[][], "Pred_Score"=w172:sgl, "NNPC_out"=w165:T31, "Distance_Matrix"=w170:variant, "dT_Predict"=w161:dbl)  [unwired: 2 in]
        "Img_Score" <- w172
        n56 = call "Combine_Anomaly_Detection_Results.vi"("Relative Resolution"=w156, "Evaluation_Results"=w150, "Display_Options"=w153, "Pixel Anomaly Thrshld"=w155, "error in"=w171, "Anomaly Map"=w173, "Gt File Path"=w185, "Orig Image In"=w157) -> ("error out"=w167:errorcluster, "Anomaly Detection Results"=w146:T65)  [unwired: 1 in, 1 out]
        n57 = call <vilib>:"Mean PtByPt.vi"("x"=w161) -> ("mean"=→"dT_Predict":dbl)  [unwired: 3 in, 1 out]
        n58 = Cluster To Array(cluster=w146) -> (array=w147:T17[])
        n59 = Unbundle By Name(w150) -> ("Threshold(Image)"=w149:sgl, "Threshold(Pixel)"=→"Pixel_Thrshld (Eval)":sgl)
        "Image_Thrshld (Eval)" <- w149
        n60 = Unbundle By Name(w146) -> ("Image"=w144:T17, "Predicted Mask"=w145:T17)
        n61 = case shown="\"CPU\", Default" w166 {
          tunnel: [w190 w198] -> w164
          tunnel: [w188 w197] -> w162
          tunnel: w170 -> [w193 w196]
          tunnel: w167 -> [w192 w195]
          frame "CPU", Default {
            n62 = Variant To Data(error in=w192, type=refnum<data-value> refnum ("data value reference"), Variant=w193) -> (data=w191:refnum<data-value>, error out=w189:errorcluster)
            n63 = call-poly <vilib>:"NN_Data_Get_ValByRef.vi"("error in (no error)"=w189, "DVR(2D_SGL)"=w191) -> ("error out"=w188:errorcluster, "Value(2D_SGL)"=w190:sgl[][])  [unwired: 6 in]
          }
          frame "GPU" {
            n64 = disable-structure shown="USE_CULAB==TRUE" {
              disable-tunnel: [w205 _] -> w198
              disable-tunnel: [w201 w206] -> w197
              disable-tunnel: w196 -> [w200 _]
              disable-tunnel: w195 -> [w199 w207]
              frame condition #0 (active) {
                n65 = Variant To Data(error in=w199, type=refnum<class "T2D_SGL.lvclass"> refnum ("Features"), Variant=w200) -> (data=w203:refnum<class "T2D_SGL.lvclass">, error out=w202:errorcluster)
                n66 = call-poly <vilib>:"CU_Tensor_Pull.vi"("error in (no error)"=w202, "T2D_SGL in"=w203) -> ("2D_SGL_Data"=w205:sgl[][], "error out"=w201:errorcluster)  [unwired: 7 in, 1 out]
              }
              frame condition #1 {
                n67 = Build Array("In order to use GPU for Patchcore, please install CuLab Toolkit and create and set conditional disable variable  with name  \"USE_CULAB\" with value \"TRUE\"." ("Message")) -> (w211:string[])
                n68 = call <vilib>:"NN_Generate_Custom_Error.vi"("show call chain? (TRUE)"=TRUE ("show call chain? (False)"), "error in (no error)"=w207, "Message"=w211, "Error_code"=403665) -> ("error out"=w206:errorcluster)  [unwired: 7 in]
              }
            }
          }
        }
        n69 = Less Than 0?(x="Image_Thrshld(Custom)") -> (x < 0?=w187:bool)
        n70 = Array Max & Min(array=w173) -> (max value=→"Pixel_Score(Max)":sgl)  [unwired: 3 out]
        n71 = Select(t=w149, s=w187, f="Image_Thrshld(Custom)") -> (s? t:f=w186:sgl)
        n72 = Greater?(x=w172, y=w186) -> (0:→"Anomaly?":bool)
      }
      event Timeout {
        w217 = u32 1 items=["Zero Order", "Bi-Linear", "Quadratic", "Cubic Spline"] ("Interpolation Type")
        n73 = event-data() -> ()  [unwired: 1 in, 1 out]
        n74 = local read "Last Mouse Position:All Elements"() -> (w274:cluster{"X":i32, "Y":i32})
        n75 = property on="Anomaly Detection Result" class="ImageControl"() -> ("Last Mouse Position"=w282:cluster{"X":i32, "Y":i32})  [unwired: 2 in, 2 out]
        n76 = Index Array(array=w267, index="Display_Image") -> (element=w260:T17)
        n77 = Select(t=w282, s="Search Mode", f=w274) -> (s? t:f=w259:cluster{"X":i32, "Y":i32})
        n78 = Divide(x=w259, y=w222) -> (x/y=w256:cluster{"X":sgl, "Y":sgl})
        n79 = To Long Integer(number=w256) -> (32bit integer=w254:cluster{"X":i32, "Y":i32})
        n80 = call "Pixel_Coords_To_Patch_Index.vi"("Selected_Coreset_Element_Info"=w240, "Coords"=w254) -> ("Flat_Patch_Coords"=w283:i32)  [unwired: 9 in]
        n81 = Index Array(array=w268, index (row)=w283) -> (element=w275:sgl[])  [unwired: 1 in]
        n82 = call "Find_Closeest_Embedding_Idx.vi"("Selected_Coreset_Element_Info"=w240, "Pixel_Thrshld(Custom)"=w241, "Distance_From_Embedding"=w275) -> ("Closest_Samples"=w284:T66[])  [unwired: 8 in]
        n83 = Array Size(array=w284) -> (size(s)=w285:i32)
        "#Closest_Samples" <- w285
        n84 = Decrement(x=w285) -> (x-1=w287:i32)
        n85 = property on="Closest_Idx" class="DigNum (strict)"("Maximum"=w287, "Minimum"=0.0 ("Data Entry Limits:Minimum")) -> ()  [unwired: 2 in, 2 out]
        n86 = Index Array(array=w284, index="Closest_Idx") -> (element=w249:T66)
        n87 = Unbundle By Name(w249) -> ("Feature_Coords"=w248:T47, "Score"=→"Closest_Score":sgl)
        n88 = Unbundle By Name("ROI Scales") -> ("Patch"=w276:sgl, "Receptive_Field"=w226:sgl)
        n89 = call "IMAQ Clear Overlay"("error in (no error)"=w265, "Image"=w260) -> ("error out"=w225:errorcluster, "Image Out"=w218:T17)  [unwired: 8 in]
        n90 = Unbundle By Name(w248) -> ("Idx"=w255:i32, "i"=w246:i32, "j"=w245:i32)
        n91 = Unbundle By Name(w220) -> ("Cropping"=w227:T20)
        n92 = Index Array(array=w270, index=w255) -> (element=w264:path)
        n93 = Unbundle By Name(w254) -> ("Y"=w263:i32, "X"=w262:i32)
        n94 = Unbundle By Name(w240) -> ("Stride"=w223:i32)
        n95 = Bundle By Name(cluster=T51 {"H"=0, "W"=0} ("Coords_In"), "H"=w246, "W"=w245) -> (w244:T51)
        n96 = call "IMAQ ReadFile"("File Path"=w264, "error in (no error)"=w225, "Image"=w266) -> ("error out"=w230:errorcluster, "Image Out"=w228:T17)  [unwired: 4 in, 3 out]
        n97 = Bundle By Name(cluster=T51 {"H"=0, "W"=0} ("Coords_Out"), "H"=w263, "W"=w262) -> (w252:T51)
        n98 = call "Img_Center_Crop.vi"("Crop_CFG"=w227, "error in"=w230, "Image Dest In"=w228, "Image Src In"=w228) -> ("error out"=w213:errorcluster, "Image Dest Out"=w216:T17)  [unwired: 6 in]
        n99 = Multiply(x=w271, y=w226) -> (x*y=w280:sgl)
        n100 = call "Coerce_and_Center_Coords.vi"("Coords_In"=w252, "Feature_Size"=w223) -> ("Coords_Out"=w251:T51)  [unwired: 5 in]
        n101 = call "Coerce_and_Center_Coords.vi"("Coords_In"=w244, "Feature_Size"=w223) -> ("Coords_Out"=w243:T51)  [unwired: 5 in]
        n102 = Multiply(x=w223, y=w276) -> (x*y=w281:sgl)
        n103 = call "IMAQ GetImageSize"("Image"=w218, "error in (no error)"=w213) -> ("Y Resolution"=w215:i32, "X Resolution"=w214:i32, "error out"=w212:errorcluster)  [unwired: 2 in]
        n104 = Build Array(w281, w280) -> (w278:sgl[])
        n105 = call "IMAQ Resample"("X Resolution"=w214, "Y Resolution"=w215, "error in (no error)"=w212, "Interpolation Type"=w217, "Image Src"=w216) -> ("error out"=w229:errorcluster, "Image Dst Out"=w219:T17)  [unwired: 5 in]
        n106 = Multiply(x=w223, y=w222) -> (x*y=w221:sgl)
        n107 = call "Pixel_Coords_to_Feature_Coords(SS).vi"("Frame_Dims"=w278, "Center_Coords"=w251) -> ("Frames"=w279:T67[])  [unwired: 9 in]
        n108 = call "Pixel_Coords_to_Feature_Coords(SS).vi"("Frame_Dims"=w278, "Center_Coords"=w243) -> ("Frames"=w286:T67[])  [unwired: 9 in]
        n109 = case shown="True" "Show Patch Grid?" {
          tunnel: w218 -> [w293 w304]
          tunnel: [w293 w303] -> w239
          tunnel: w225 -> [w292 w302]
          tunnel: w221 -> [_ w301]
          tunnel: w219 -> [w294 w300]
          tunnel: [w294 w299] -> w234
          tunnel: [w291 w296] -> w238
          tunnel: w229 -> [w291 w298]
          tunnel: [w292 w295] -> w235
          frame False {
          }
          frame True {
            w297 = u32 6618880 ("Grid Color")
            n110 = call "Draw_Grid.vi"("Grid Color"=w297, "error in (no error)"=w302, "Grid_Size"=w301, "Image_In"=w304) -> ("error out"=w295:errorcluster, "Image_Out"=w303:T17)  [unwired: 6 in]
            n111 = call "Draw_Grid.vi"("Grid Color"=w297, "error in (no error)"=w298, "Grid_Size"=w301, "Image_In"=w300) -> ("error out"=w296:errorcluster, "Image_Out"=w299:T17)  [unwired: 6 in]
          }
        }
        n112 = Multiply(x=w279, y=w222) -> (x*y=w257:T67[])
        n113 = Multiply(x=w286, y=w222) -> (x*y=w258:T67[])
        n114 = for {
          tunnel: "Feature Color" -> [w311]
          tunnel: w257 -> [w310] mode=indexing
          tunnel: w235 -> [w309]
          shift-right: [w307] -> w237
          shift-left: w239 -> [w308]
          tunnel: [w305] -> w233
          stop <- w305 stop-if-true
          w306 = u32 0 items=["Frame", "Fill"] ("Drawing Mode (Frame)")
          n115 = call "IMAQ Overlay Rectangle"("Color"=w311, "error in (no error)"=w309, "Drawing Mode (Frame)"=w306, "Rectangle"=w310, "Image"=w308) -> ("error out"=w305:errorcluster, "Image Out"=w307:T17)  [unwired: 5 in]
        }
        "Anomaly Detection Result" <- w237
        n116 = for {
          tunnel: "Feature Color" -> [w318]
          tunnel: w258 -> [w317] mode=indexing
          shift-right: [w314] -> w236
          shift-left: w234 -> [w316]
          tunnel: w238 -> [w315]
          tunnel: [w312] -> w232
          stop <- w312 stop-if-true
          w313 = u32 0 items=["Frame", "Fill"] ("Drawing Mode (Frame)")
          n117 = call "IMAQ Overlay Rectangle"("Color"=w318, "error in (no error)"=w315, "Drawing Mode (Frame)"=w313, "Rectangle"=w317, "Image"=w316) -> ("error out"=w312:errorcluster, "Image Out"=w314:T17)  [unwired: 5 in]
        }
        "Closest_Train_Sample" <- w236
        n118 = Merge Errors(w233, w232) -> (w231:errorcluster)
      }
      event "Anomaly Detection Result": Mouse Down {
        n119 = event-data() -> ()  [unwired: 1 in, 1 out]
        n120 = property on="Anomaly Detection Result" class="ImageControl"(error in=w324) -> (error out=w323:errorcluster, "Last Mouse Position"=→"Last Mouse Position:All Elements":cluster{"X":i32, "Y":i32})  [unwired: 1 in, 1 out]
      }
      event "DS Selector": Value Change {
        n121 = event-data() -> ("NewVal"=w335:enum16{"Good", "Bad", "Both"})  [unwired: 1 in]
        n122 = local read "Order"() -> (w331:enum16{"Ascending", "Descending", "File"})
        n123 = case shown="\"Good\", Default" w335 {
          tunnel: w334 -> [w336 _ w340]
          tunnel: w333 -> [_ w337 w339]
          tunnel: [w336 w337 w338] -> w332
          frame "Good", Default {
          }
          frame "Bad" {
          }
          frame "Both" {
            n124 = Build Array (concatenate)(w340, w339) -> (w338:T24[])
          }
        }
        n125 = property on="Order" class="Enum (strict)"(error in=w330, "Val(Sgnl)"=w331) -> (error out=w329:errorcluster)  [unwired: 1 in, 1 out]
      }
      event "Order": Value Change {
        w349 = u32 0 ("Data Entry Limits:Minimum")
        n126 = event-data() -> ("NewVal"=w354:enum16{"Ascending", "Descending", "File"})  [unwired: 1 in]
        n127 = case shown="\"Ascending\", Default" w354 {
          tunnel: [w355 w371 w384] -> w351
          tunnel: w353 -> [w357 w370 w384]
          frame "Ascending", Default {
            n128 = for {
              tunnel: w357 -> [w366] mode=indexing
              tunnel: [w365] -> w359 mode=indexing
              i -> [w364]
              n129 = Unbundle By Name(w366) -> ("Image Score"=w363:sgl)
              n130 = Bundle("Image Score"=w363, w364) -> (w365:cluster{"Image Score":sgl, i32})  [unwired: 1 in]
            }
            n131 = Sort 1D Array(array=w359) -> (sorted array=w358:cluster{"Image Score":sgl, i32}[])
            n132 = for {
              tunnel: w358 -> [w368] mode=indexing
              tunnel: [w367] -> w356 mode=indexing
              n133 = Unbundle(w368) -> (w367:i32)  [unwired: 1 out]
            }
            n134 = for {
              tunnel: w357 -> [w362]
              tunnel: w356 -> [w361] mode=indexing
              tunnel: [w360] -> w355 mode=indexing
              n135 = Index Array(array=w362, index=w361) -> (element=w360:T24)
            }
          }
          frame "Descending" {
            n136 = for {
              tunnel: w370 -> [w381] mode=indexing
              tunnel: [w380] -> w372 mode=indexing
              i -> [w379]
              n137 = Unbundle By Name(w381) -> ("Image Score"=w378:sgl)
              n138 = Bundle("Image Score"=w378, w379) -> (w380:cluster{"Image Score":sgl, i32})  [unwired: 1 in]
            }
            n139 = Sort 1D Array(array=w372) -> (sorted array=w373:cluster{"Image Score":sgl, i32}[])
            n140 = Reverse 1D Array(array=w373) -> (reversed array=w369:cluster{"Image Score":sgl, i32}[])
            n141 = for {
              tunnel: w369 -> [w383] mode=indexing
              tunnel: [w382] -> w374 mode=indexing
              n142 = Unbundle(w383) -> (w382:i32)  [unwired: 1 out]
            }
            n143 = for {
              tunnel: w370 -> [w377]
              tunnel: w374 -> [w376] mode=indexing
              tunnel: [w375] -> w371 mode=indexing
              n144 = Index Array(array=w377, index=w376) -> (element=w375:T24)
            }
          }
          frame "File" {
          }
        }
        n145 = local read "index"() -> (w347:i32)
        n146 = property on="index" class="DigNum (strict)"(error in=w346, "Val(Sgnl)"=w347) -> (error out=w345:errorcluster)  [unwired: 1 in, 1 out]
        n147 = Array Size(array=w351) -> (size(s)=w350:i32)
        n148 = Decrement(x=w350) -> (x-1=w352:i32)
        n149 = property on="index" class="DigNum (strict)"(error in=w345, "Maximum"=w352, "Minimum"=w349, "OutOfRngActMax"=u8 1 ("Response to Value Outside Limits:Maximum"), "OutOfRngActMin"=w349) -> (error out=w344:errorcluster)  [unwired: 1 in, 1 out]
      }
    }
    n150 = Or(x=w126, y=w127) -> (x .or. y?=w137:bool)
  }
  n151 = Build Array(w2) -> (w1:T29[])
  n152 = call <vilib>:"NNPC_Destroy.vi"("Datasets_to_Destroy"=w1, "error in"=w18, "NNPC_in"=w20) -> ("error out"=→"error out":errorcluster)  [unwired: 8 in]
